vi "MicrotimeMain.vi"() -> ()   [LabVIEW 2013]
uses:
  <vilib>/vision/Pattern Matching.llb/IMAQ Curve Parameters.ctl
  <vilib>/vision/Pattern Matching.llb/IMAQ Match Range Setting.ctl
  <vilib>/vision/Image Controls.llb/IMAQ Rounding Mode.ctl
  Camera/lib/System Files/user.lib/atmcd32d.llb/Shutter_type typedef.ctl
  Camera/lib/System Files/user.lib/atmcd32d.llb/Shutter_mode typedef.ctl
  Variables/patternImg.vi
  Camera/vi/GlobalSetGetConfigureCamera.vi
  Camera/vi/ccdChipPixels.vi
  Variables/GetPicture.vi
  Variables/GlobalConAxisPI.vi
  Variables/GlobalLaserInterface.vi
  Camera/vi/StopGetPic.vi
  Camera/vi/CamDef.vi
  Camera/lib/System Files/user.lib/atmcd32d.llb/Error Code Enum typedef.ctl
panel:
  out "subarray":dbl[](array[numeric])
  in  "Settings (GeometricMatching)":T3={"Curve Parameters"={"Extraction Mode"=0, "Edge Threshold"=75, "Edge Filter Size"=1, "Min Length"=25, "Row Search Step Size"=15, "Col Search Step Size"=15, "Max Endpoint Gap"=10, "Closed"=FALSE, "Subpixel"=FALSE}, "Match Mode"={"Rotation"=TRUE, "Scale"=FALSE, "Occlusion"=TRUE, "Reserved"=FALSE, "Reserved"=FALSE, "Reserved"=FALSE}, "Range Settings"=[{"Match Constraints"=0, "Min"=0.0, "Max"=360.0}, {"Match Constraints"=2, "Min"=0.0, "Max"=25.0}], "Number of Matches"=5, "Minimum Match Score"=600.0, "SubPixel Accuracy"=FALSE, "Adv. Geometric Match Options 2"=[{"Setup Data Item"=21, "Item Value"=0.0}, {"Setup Data Item"=22, "Item Value"=1.0}]} {"Curve Parameters"."Extraction Mode" items=["Normal", "Uniform Regions"]; "Curve Parameters"."Edge Filter Size" items=["Fine", "Normal", "Contour Tracing"]; "Curve Parameters"."Max Endpoint Gap" min=0; "Curve Parameters"."Col Search Step Size" min=1 max=255 step=1; "Curve Parameters"."Row Search Step Size" min=1 max=255 step=1; "Curve Parameters"."Min Length" min=0; "Curve Parameters"."Edge Threshold" min=1 max=350 step=1; "Range Settings"."Max" format="%.2f"; "Range Settings"."Min" format="%.2f"; "Range Settings"."Match Constraints" items=["Rotation Angle (degrees)", "Scale Factor (%)", "Occlusion (%)"]; "Adv. Geometric Match Options 2"."Setup Data Item" items=["Curve Extraction Mode", "Curve Edge Threshold", "Curve Edge Filter Size", "Min Curve Length", "Curve Row Search Step Size", "Curve Col Search Step Size", "Curve Max Endpoint Gap", "Extract Closed Curves", "Enable Subpixel Curve Extraction", "Enable Correlation Score", "Enable Subpixel Accuracy", "Subpixel Iterations", "Subpixel Tolerance", "Initial Match List Length", "Enable Target Template Curve Score", "Min Match Separation Distance", "Min Match Separation Angle", "Min Match Separation Scale", "Max Match Overlap", "Enable Coarse Result", "Enable Calibration Support", "Enable Contrast Reversal", "Search Strategy", "Refinement Match Factor", "Subpixel Match Factor"]}
  in  "Tab Control":T4(tab)
  out "Histogram":i32[][](graph)
  out "Trace":i32[][](graph)=[[2, 0, 0, 1, 1, 1, 0, 0, 0, 1, 0, 1, 0, 1, 2, 2, 0, 3, 0, 2, 2, 1, 3, 1, 0, 1, 1, 1, 0, 1, 3, 1, 0, 2, 0, 1, 0, 1, 1, 0, 1, 1, 3, 1, 0, 2, 0, 1, 1, 0, 0, 2, 0, 0, 1, 1, 1, 0, 0, 1, 0, 1, 0, 0, 0, 1, 2, 1, 1, 2, 0, 2, 4, 3, 1, 1, 0, 0, 1, 1, 2, 0, 1, 1, 0, 0, 0, 1, 1, 1, 1, 3, 0, 0, 1, 0, 0, 0, 2, 1, 1, 1, 2, 1, 0, 1, 1, 0, 0, 2, 1, 1, 0, 0, 1, 1, 1, 1, 0, 2, 2, 0, 1, 2, 1, 0, 3, 0, 2, 1, 3, 0, 1, 1, 0, 0, 3, 0, 0, 0, 0, 0, 0, 0, 0, 0, 0, 0, 0, 0, 0, 0, 0, 0, 0, 0, 0, 0, 0, 0, 0, 0, 0, 0, 0, 0, 0, 0, 0, 0, 0, 0, 0, 0, 0, 0, 0, 0, 0, 0, 0, 0, 0, 0, 0, 0, 0, 0, 0, 0, 0, 0, 0, 0, 0, 0, 0, 0, 0, 0], [1, 2, 2, 0, 0, 0, 1, 2, 1, 2, 1, 1, 1, 0, 0, 0, 3, 1, 0, 1, 0, 2, 0, 2, 1, 1, 0, 0, 1, 0, 1, 2, 1, 0, 0, 0, 0, 0, 1, 0, 1, 0, 2, 0, 1, 0, 0, 0, 0, 1, 1, 3, 0, 0, 0, 2, 0, 0, 2, 0, 1, 1, 0, 0, 2, 0, 2, 1, 0, 1, 1, 0, 1, 1, 0, 0, 0, 1, 0, 0, 1, 0, 0, 0, 0, 1, 0, 1, 1, 1, 1, 0, 0, 0, 1, 1, 1, 0, 1, 0, 0, 0, 1, 1, 1, 0, 0, 1, 1, 3, 1, 0, 0, 0, 0, 0, 0, 0, 1, 2, 1, 0, 0, 0, 2, 3, 3, 2, 0, 1, 1, 1, 0, 0, 4, 0, 1, 2, 0, 0, 0, 2, 0, 0, 0, 0, 0, 0, 0, 0, 0, 0, 0, 0, 0, 0, 0, 0, 0, 0, 0, 0, 0, 0, 0, 0, 0, 0, 0, 0, 0, 0, 0, 0, 0, 0, 0, 0, 0, 0, 0, 0, 0, 0, 0, 0, 0, 0, 0, 0, 0, 0, 0, 0, 0, 0, 0, 0, 0, 0], [2, 2, 0, 1, 2, 0, 1, 0, 2, 3, 1, 0, 1, 0, 1, 0, 0, 0, 0, 2, 1, 0, 0, 2, 2, 0, 0, 0, 3, 0, 0, 2, 2, 2, 0, 3, 0, 3, 1, 3, 1, 3, 1, 0, 3, 1, 3, 3, 1, 1, 1, 1, 2, 0, 1, 0, 1, 1, 1, 3, 0, 2, 3, 1, 1, 1, 0, 1, 0, 1, 2, 3, 1, 2, 1, 3, 0, 2, 0, 2, 0, 1, 0, 2, 2, 1, 1, 3, 1, 2, 1, 1, 1, 3, 0, 0, 0, 0, 1, 1, 1, 0, 1, 0, 2, 1, 1, 0, 1, 0, 1, 2, 2, 2, 2, 0, 1, 0, 0, 0, 1, 1, 2, 0, 0, 1, 5, 2, 2, 0, 2, 0, 2, 2, 2, 0, 1, 0, 6, 0, 0, 0, 0, 0, 0, 0, 0, 0, 0, 0, 0, 0, 0, 0, 0, 0, 0, 0, 0, 0, 0, 0, 0, 0, 0, 0, 0, 0, 0, 0, 0, 0, 0, 0, 0, 0, 0, 0, 0, 0, 0, 0, 0, 0, 0, 0, 0, 0, 0, 0, 0, 0, 0, 0, 0, 0, 0, 0, 0, 0], [0, 0, 1, 0, 1, 1, 0, 0, 0, 1, 1, 0, 1, 0, 0, 0, 0, 0, 2, 0, 0, 0, 0, 2, 0, 0, 0, 1, 1, 2, 1, 1, 1, 2, 1, 0, 0, 3, 0, 1, 1, 0, 0, 0, 0, 1, 0, 0, 2, 1, 0, 0, 1, 1, 1, 2, 2, 0, 1, 0, 0, 1, 0, 1, 1, 0, 0, 2, 1, 1, 2, 1, 1, 0, 0, 0, 0, 2, 1, 0, 0, 0, 0, 1, 0, 1, 0, 0, 0, 0, 1, 0, 0, 0, 0, 1, 0, 1, 1, 1, 0, 2, 3, 1, 1, 0, 1, 1, 1, 0, 1, 0, 0, 1, 1, 0, 2, 0, 0, 0, 0, 3, 0, 0, 0, 0, 0, 0, 0, 0, 1, 0, 2, 0, 0, 0, 1, 2, 2, 0, 1, 0, 0, 0, 0, 0, 0, 0, 0, 0, 0, 0, 0, 0, 0, 0, 0, 0, 0, 0, 0, 0, 0, 0, 0, 0, 0, 0, 0, 0, 0, 0, 0, 0, 0, 0, 0, 0, 0, 0, 0, 0, 0, 0, 0, 0, 0, 0, 0, 0, 0, 0, 0, 0, 0, 0, 0, 0, 0, 0]]
  out "CCD":i32[][](graph)
  out "Image Out":T5(plugin-control)
  out "Image Number":u32
  out "acquired FPS":dbl
  out "Image":i32[][](graph)
  out "AM image":T5(plugin-control)
  out "Number of Particles":i32
  out "Auto Measure Points":i32
  out "NxtAutMesPoint":i32
  out "Pattern":dbl[][](array[numeric])
  out "X Steps":dbl
  out "3dAbelFcs":bool=TRUE
  out "Y Steps":dbl
  out "Z Steps":dbl
  out "concatenated string":string
  out "Global Stop":bool=TRUE
  out "Stop Measurement":bool
  in  "DeviceTabs":T6(tab)
  in  "WS File Tree":string(tree)
  out "Workspace":path=path "X:/MTusers/Christoph/2011-02-01 Andi/2011-02-01.msw"
  in  "New MSW":bool
  in  "Open MSW":bool
  in  "Sample description":string
  in  "Save Files":bool=TRUE
  out "Last Image File No":i32=-1
  in  "Get Position":bool
  in  "Move Stage":bool
  in  "X-Position":dbl=48.0021 caption="X" min=0.0 max=200.0 step=0.1 format="%1.3f um"
  in  "Y-Position":dbl=19.9997 caption="Y" min=0.0 max=200.0 step=0.1 format="%1.3f um"
  in  "Z-Position":dbl=69.999 caption="Z" min=0.0 max=200.0 step=0.1 format="%1.3f um"
  out "x-position":dbl format="%.3f"
  out "y-position":dbl format="%.3f"
  out "z-position":dbl format="%.3f"
  in  "CFD Settings":T7={"Sync Level"=15, "Sync ZeroX"=0, "Sync Offset"=0, "Chan Settings"=[{"CHx Level"=50, "CHx ZeroX"=10, "CHx Offset"=-22150}, {"CHx Level"=50, "CHx ZeroX"=10, "CHx Offset"=-21850}, {"CHx Level"=75, "CHx ZeroX"=10, "CHx Offset"=-6000}, {"CHx Level"=75, "CHx ZeroX"=10, "CHx Offset"=-5700}]}
  in  "Laser  Profile":string="1"
  in  "Auto Exposure::Mode":u32(ring) items=["Relative"=0, "Ignored"=5]
  in  "Brightness::Mode":u32(ring) items=["Relative"=0, "Ignored"=5]
  in  "Gain::Mode":u32(ring) items=["Absolute"=1, "Auto"=3, "Relative"=0, "Ignored"=5]
  in  "Gamma::Mode":u32(ring)=2 items=["Relative"=0, "Off"=2, "Ignored"=5]
  in  "Shutter::Mode":u32(ring) items=["Auto"=3, "Relative"=0, "Ignored"=5]
  in  "Trigger::Trigger Activation":u32(ring) items=["Level Low", "Level High"]
  in  "Trigger::Trigger Mode":u32(ring)=16 items=["Mode 0"=0, "Mode 1"=1, "Mode 15"=15, "Off"=16]
  in  "Trigger Delay::Mode":u32(ring)=2 items=["Absolute"=1, "Relative"=0, "Off"=2, "Ignored"=5]
  in  "Brightness::Value":dbl=16.0 min=0.0 max=1023.0 step=1.0
  in  "Shutter::Value":dbl=436.0 min=1.0 max=4095.0 step=1.0
  in  "Auto Exposure::Value":dbl=125.0 min=50.0 max=205.0 step=1.0
  in  "Gain::Value":dbl min=0.0 max=680.0 step=1.0
  in  "Trigger::Trigger Parameter":u32 max=0
  in  "Get Temperature":bool
  in  "SET CCD":bool
  in  "OPEN SHUTER":bool
  in  "Close":bool
  in  "Gain":bool
  in  "Start":bool
  in  "Stop":bool
  in  "Exposure":bool
  in  "Set Temperature":bool
  in  "PI SystemNumber":i32=1
  in  "Image Measurent Parameters":T8
  in  "Measurement Tab Control":T9(tab)
  in  "SCANNER EMERGENCY":bool
  in  "Stop Program":bool
  out "Task":T10(ring)
  in  "Point Defocussed Cam":bool
  in  "Adjustment":bool
  in  "Laser pulse duration":i32[](array[numeric]) min=2 max=100000 step=1 format="%d µs"
  in  "Measurement Time":i32=60 min=10 format="%.0d s"
  in  "Point Measurement":bool
  out "Counts":u32[](array[numeric])
  in  "Axis":enum32{"x-y", "x-z", "y-x", "y-z", "z-x", "z-y"}(ring)
  in  "Picture size 2":dbl=50.0 min=0.1 max=200.0 format="%1.1f um"
  in  "Picture size":dbl=50.0 min=0.1 max=200.0 format="%1.1f um"
  in  "Pixel time":dbl=1.0 min=0.1 max=10.0 step=0.1 format="%.1f ms"
  in  "Resolution":dbl=1.0 min=0.05 max=10.0 step=0.05 format="%.2f µm"
  out "Measure. time":dbl format="%7.1f s"
  in  "Aquire Image":bool
  out "y":i16=500
  out "x":i16=500
  in  "Save Color Image":bool
  in  "Cam (Defocused)":bool
  in  "How long?":bool
  out "Estimated Time (h)":dbl
  in  "Mesaurement Time (Sec) / Step":dbl
  in  "Start 3D FCS Abel Scan":bool
  in  "FCS Point Measurement":bool
  in  "Z Stepsize":dbl
  in  "Y Stepsize":dbl
  in  "X Stepsize":dbl
  in  "Z End":dbl
  in  "Y End":dbl
  in  "X End":dbl
  in  "Z Start":dbl
  in  "Y Start":dbl
  in  "X Start":dbl
  in  "Manual":bool
  in  "Find Mols":bool
  in  "Filter":bool=TRUE
  in  "Remove Outliers":i32=10
  in  "Exclude / Include X":bool
  in  "X Start 2":dbl
  in  "X End 2":dbl
  in  "Exclude / Include Y":bool
  in  "Y Start 2":dbl
  in  "Y End 2":dbl
  in  "Measurement Parameter 1":T11 items=["Center of Mass X", "Center of Mass Y", "First Pixel X", "First Pixel Y", "Bounding Rect Left", "Bounding Rect Top", "Bounding Rect Right", "Bounding Rect Bottom", "Max Feret Diameter Start X", "Max Feret Diameter Start Y", "Max Feret Diameter End X", "Max Feret Diameter End Y", "Max Horiz. Segment Length Left", "Max Horiz. Segment Length Right", "Max Horiz. Segment Length Row", "-", "Bounding Rect Width", "Bounding Rect Height", "Bounding Rect Diagonal", "Perimeter", "Convex Hull Perimeter", "Holes' Perimeter", "Max Feret Diameter", "Equivalent Ellipse Major Axis", "Equivalent Ellipse Minor Axis", "Equivalent Ellipse Minor Axis (Feret)", "Equivalent Rect Long Side", "Equivalent Rect Short Side", "Equivalent Rect Diagonal", "Equivalent Rect Short Side (Feret)", "Average Horiz. Segment Length", "Average Vert. Segment Length", "Hydraulic Radius", "Waddel Disk Diameter", "-", "Area", "Holes' Area", "Particle & Holes' Area", "Convex Hull Area", "Image Area", "-", "Number of Holes", "Number of Horiz. Segments", "Number of Vert. Segments", "-", "Orientation", "Max Feret Diameter Orientation", "-", "% Area/Image Area", "% Area/(Particle & Holes' Area)", "Ratio of Equivalent Ellipse Axes", "Ratio of Equivalent Rect Sides", "-", "Elongation Factor", "Compactness Factor", "Heywood Circularity Factor", "Type Factor", "-", "Sum X", "Sum Y", "Sum XX", "Sum XY", "Sum YY", "Sum XXX", "Sum XXY", "Sum XYY", "Sum YYY", "-", "Moment of Inertia XX", "Moment of Inertia XY", "Moment of Inertia YY", "Moment of Inertia XXX", "Moment of Inertia XXY", "Moment of Inertia XYY", "Moment of Inertia YYY", "Norm. Moment of Inertia XX", "Norm. Moment of Inertia XY", "Norm. Moment of Inertia YY", "Norm. Moment of Inertia XXX", "Norm. Moment of Inertia XXY", "Norm. Moment of Inertia XYY", "Norm. Moment of Inertia YYY", "Hu Moment 1", "Hu Moment 2", "Hu Moment 3", "Hu Moment 4", "Hu Moment 5", "Hu Moment 6", "Hu Moment 7"]
  in  "Range Lower Value Par 1":dbl
  in  "Range Upper Value  Par 1":dbl
  in  "Ex/In Par 1":bool
  in  "Measurement Parameter 2":T11 items=["Center of Mass X", "Center of Mass Y", "First Pixel X", "First Pixel Y", "Bounding Rect Left", "Bounding Rect Top", "Bounding Rect Right", "Bounding Rect Bottom", "Max Feret Diameter Start X", "Max Feret Diameter Start Y", "Max Feret Diameter End X", "Max Feret Diameter End Y", "Max Horiz. Segment Length Left", "Max Horiz. Segment Length Right", "Max Horiz. Segment Length Row", "-", "Bounding Rect Width", "Bounding Rect Height", "Bounding Rect Diagonal", "Perimeter", "Convex Hull Perimeter", "Holes' Perimeter", "Max Feret Diameter", "Equivalent Ellipse Major Axis", "Equivalent Ellipse Minor Axis", "Equivalent Ellipse Minor Axis (Feret)", "Equivalent Rect Long Side", "Equivalent Rect Short Side", "Equivalent Rect Diagonal", "Equivalent Rect Short Side (Feret)", "Average Horiz. Segment Length", "Average Vert. Segment Length", "Hydraulic Radius", "Waddel Disk Diameter", "-", "Area", "Holes' Area", "Particle & Holes' Area", "Convex Hull Area", "Image Area", "-", "Number of Holes", "Number of Horiz. Segments", "Number of Vert. Segments", "-", "Orientation", "Max Feret Diameter Orientation", "-", "% Area/Image Area", "% Area/(Particle & Holes' Area)", "Ratio of Equivalent Ellipse Axes", "Ratio of Equivalent Rect Sides", "-", "Elongation Factor", "Compactness Factor", "Heywood Circularity Factor", "Type Factor", "-", "Sum X", "Sum Y", "Sum XX", "Sum XY", "Sum YY", "Sum XXX", "Sum XXY", "Sum XYY", "Sum YYY", "-", "Moment of Inertia XX", "Moment of Inertia XY", "Moment of Inertia YY", "Moment of Inertia XXX", "Moment of Inertia XXY", "Moment of Inertia XYY", "Moment of Inertia YYY", "Norm. Moment of Inertia XX", "Norm. Moment of Inertia XY", "Norm. Moment of Inertia YY", "Norm. Moment of Inertia XXX", "Norm. Moment of Inertia XXY", "Norm. Moment of Inertia XYY", "Norm. Moment of Inertia YYY", "Hu Moment 1", "Hu Moment 2", "Hu Moment 3", "Hu Moment 4", "Hu Moment 5", "Hu Moment 6", "Hu Moment 7"]
  in  "Range Lower Value Par 2":dbl
  in  "Range Upper Value Par 2":dbl
  in  "Ex/In Par 2":bool
  in  "Square/Hexa":bool=TRUE
  in  "Connectivity 4/8":bool
  in  "Auto Defocussed Cam":bool
  in  "Autopoint-Autofocus Z":bool=TRUE
  in  "Auto Measurement Time (ms)":i32=60 caption="Measurement Time (s)" min=10
  out "Auto Meas Progress":i32(slide) caption="Point 2 / 2" scale=0.0..2.0
  in  "Auto Meas":bool
  out "Active pt3":path
  out "Buffer Overrun":bool
  out "Running":bool
  # "Range"
  # "Scanner Position"
  # "Point Measurement Settings"
  # "Start Experiment"
  # "Estimated Mesaurement Time"
  # "Image Scan Settings"
  # "Save as png"
  # "Pixel"
  # "Define the 3D Space and Stepwith of your Experiment"
  # "Time of the Experiment"
  # "Check What to Mesaure"
  # "Start Your Experiment here"
  # "Lifetime Mesaurement Time on each Position"
  # "Define Search Area"
  # "Define Detection Parameters"
  # "Exact Matching"
  # "Show Progress"
  # "Automated Mesaurement on Single Molecule Coordinates on the  2D Frame"
  # "Start Your Experiment here"
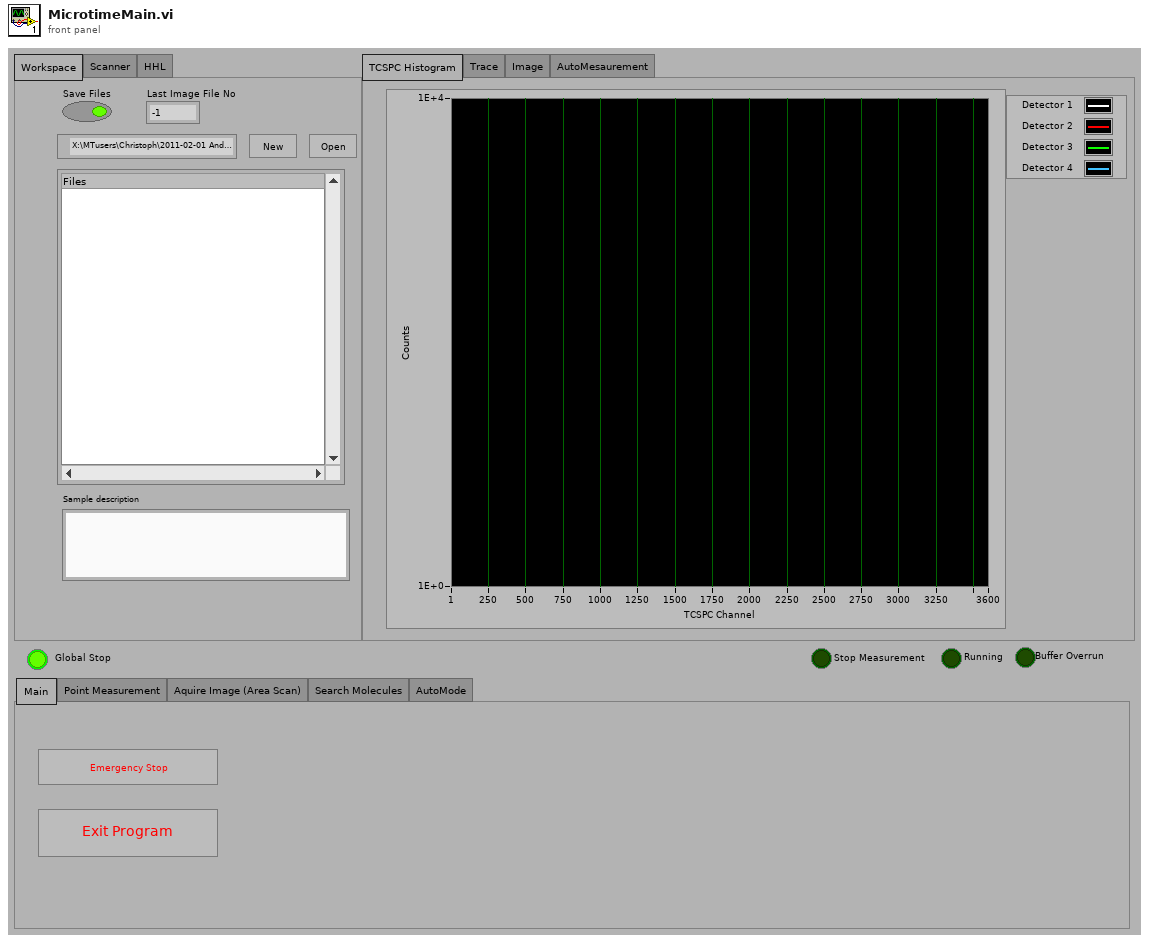
[diagram p1: front panel]
types:
  T1 = typedef "IMAQ Curve Parameters.ctl" = cluster{"Extraction Mode":u32, "Edge Threshold":i32, "Edge Filter Size":u32, "Min Length":i32, "Row Search Step Size":i32, "Col Search Step Size":i32, "Max Endpoint Gap":i32, "Closed":bool, "Subpixel":bool}
  T2 = typedef "IMAQ Match Range Setting.ctl" = cluster{"Match Constraints":u32, "Min":dbl, "Max":dbl}
  T3 = cluster{"Curve Parameters":T1, "Match Mode":cluster{"Rotation":bool, "Scale":bool, "Occlusion":bool, "Reserved":bool, "Reserved":bool, "Reserved":bool}, "Range Settings":T2[], "Number of Matches":i32, "Minimum Match Score":sgl, "SubPixel Accuracy":bool, "Adv. Geometric Match Options 2":cluster{"Setup Data Item":u16, "Item Value":dbl}[]}
  T4 = enum32{"TCSPC Histogram", "Trace", "CCD", "Backreflection", "Image", "AutoMesaurement"}
  T5 = typedef "IMAQ Image.ctl" = refnum<image>
  T6 = enum32{"Workspace", "Scanner", "HHL", "Video", "CCD"}
  T7 = cluster{"Sync Level":i32, "Sync ZeroX":i32, "Sync Offset":i32, "Chan Settings":cluster{"CHx Level":i32, "CHx ZeroX":i32, "CHx Offset":i32}[]}
  T8 = cluster{"Position":cluster{"X-Position":dbl, "Y-Position":dbl, "Z-Position":dbl}, "Axis 1 Pixels":dbl, "Axis 2 Pixels":dbl, "Axis":i32, "Resolution":dbl, "PixelTime":dbl, "Laser pulses":i32}
  T9 = enum32{"Main ", "Point Measurement", "Aquire Image (Area Scan)", "3D Grid FCS CCD", "Search Molecules", "AutoMode"}
  T10 = enum16{"No Measurement", "Aquire Image", "Point Measurement", "Multi Measurement", "Save Color Image", "Find Single Mol.", "Auto Measurement Control", "Auto Point", "Aquire Line Scan", "Grid Measurement", "Trapping", "Move Scanner"}
  T11 = typedef "Particle Parameters" = i32
  T12 = cluster{"Dev":i32, "SerNo":string, "HW_Model":string, "HW_Partno":string}[]
  T13 = typedef "Shutter_type typedef.ctl" = enum16{"TTL Low", "TTL High"}
  T14 = typedef "Shutter_mode typedef.ctl" = enum16{"Auto", "Open", "Close"}
  T15 = typedef "Error Code Enum typedef.ctl" = enum32{"N/A (0)", "DRV_ERROR_CODES", "DRV_SUCCESS", "DRV_VXDNOTINSTALLED", "DRV_ERROR_SCAN", "DRV_ERROR_CHECK_SUM", "DRV_ERROR_FILELOAD", "DRV_UNKNOWN_FUNC", "DRV_ERROR_VXD_INIT", "DRV_ERROR_ADDRESS", "DRV_ERROR_PAGELOCK", "DRV_ERROR_PAGEUNLOCK", "DRV_ERROR_BOARDTEST", "DRV_ERROR_ACK", "DRV_ERROR_UP_FIFO", "DRV_ERROR_PATTERN", "N/A (16)", "DRV_ACQUISITION_ERRORS", "DRV_ACQ_BUFFER", "DRV_ACQ_DOWNFIFO_FULL", "DRV_PROC_UNKONWN_INSTRUCTION", "DRV_ILLEGAL_OP_CODE", "DRV_KINETIC_TIME_NOT_MET", "DRV_ACCUM_TIME_NOT_MET", "DRV_NO_NEW_DATA", "N/A (25)", "DRV_SPOOLERROR", "N/A (27)", "N/A (28)", "N/A (29)", "N/A (30)", "N/A (31)", "N/A (32)", "DRV_TEMPERATURE_CODES", "DRV_TEMPERATURE_OFF", "DRV_TEMPERATURE_NOT_STABILIZED", "DRV_TEMPERATURE_STABILIZED", "DRV_TEMPERATURE_NOT_REACHED", "DRV_TEMPERATURE_OUT_RANGE", "DRV_TEMPERATURE_NOT_SUPPORTED", "DRV_TEMPERATURE_DRIFT", "N/A (41)", "N/A (42)", "N/A (43)", "N/A (44)", "N/A (45)", "N/A (46)", "N/A (47)", "N/A (48)", "DRV_GENERAL_ERRORS", "DRV_INVALID_AUX", "DRV_COF_NOTLOADED", "DRV_FPGAPROG", "DRV_FLEXERROR", "DRV_GPIBERROR", "N/A (55)", "N/A (56)", "N/A (57)", "N/A (58)", "N/A (59)", "N/A (60)", "N/A (61)", "N/A (62)", "N/A (63)", "DRV_DATATYPE", "DRV_DRIVER_ERRORS", "DRV_P1INVALID", "DRV_P2INVALID", "DRV_P3INVALID", "DRV_P4INVALID", "DRV_INIERROR", "DRV_COFERROR", "DRV_ACQUIRING", "DRV_IDLE", "DRV_TEMPCYCLE", "DRV_NOT_INITIALIZED", "DRV_P5INVALID", "DRV_P6INVALID", "DRV_INVALID_MODE", "DRV_INVALID_FILTER", "DRV_I2CERRORS", "DRV_I2CDEVNOTFOUND", "DRV_I2CTIMEOUT", "DRV_P7INVALID", "N/A (84)", "N/A (85)", "N/A (86)", "N/A (87)", "N/A (88)", "N/A (89)", "DRV_IOCERROR", "DRV_VRMVERSIONERROR"}
  T16 = cluster{"X-Position":dbl, "Y-Position":dbl, "Z-Position":dbl}
  T17 = enum16{"No Measurement", "Aquire Image", "Point Measurement", "Multi Measurement", "Save Color Image"}
  T18 = enum16{"No Measurement", "Aquire Image", "Point Measurement", "Multi Measurement", "Save Color Image", "Find Single Mol.", "Auto Measurement Control", "Auto Point"}
  T19 = enum16{"No Measurement", "Aquire Image", "Point Measurement", "Multi Measurement", "Save Color Image", "Find Single Mol."}
  T20 = enum16{"Get (Default)", "Set Workspace", "Append File", "Change Comment"}
  T21 = cluster{"File No":i32, "File Path":path, "Parent File":i32, "File Type":enum16{"unknown", "pt3 File", "png Image", "bmp Image"}, "Measurement Type":enum16{"not a pt3 File", "Image File", "Point Measurement", "Auto Point", "Line Scan", "Grid Scan"}, "Upper Left":cluster{"x-Position":dbl, "y-Position":dbl, "z-Position":dbl}, "Pixels":dbl[], "Resolution":dbl, "Scan Axis":enum32{"x-y", "x-z", "y-x", "y-z", "z-x", "z-y"}, "PixelTime":dbl}[]
  T22 = cluster{"File No":i32, "File Path":path, "Parent File":i32, "File Type":enum16{"unknown", "pt3 File", "png Image", "bmp Image"}, "Measurement Type":enum16{"not a pt3 File", "Image File", "Point Measurement", "Auto Point", "Line Scan", "Grid Scan"}, "Upper Left":cluster{"x-Position":dbl, "y-Position":dbl, "z-Position":dbl}, "Pixels":i32[], "Scan Axis":enum32{"x-y", "x-z", "y-x", "y-z", "z-x", "z-y"}, "Resolution":dbl, "PixelTime":dbl}[]
  T23 = cluster{"File No":i32, "File Path":path, "Parent File":i32, "File Type":enum16{"unknown", "pt3 File", "png Image", "bmp Image"}, "Measurement Type":enum16{"not a pt3 File", "Image File", "Point Measurement", "Auto Point", "Line Scan", "Grid Scan"}, "Upper Left":cluster{"x-Position":dbl, "y-Position":dbl, "z-Position":dbl}, "Pixels":i32[], "Resolution":dbl, "Scan Axis":enum32{"x-y", "x-z", "y-z"}, "PixelTime":dbl}[]
  T24 = cluster{"Files in Workspace[0]":cluster{"File No":i32, "File Path":path, "Parent File":i32, "File Type":enum16{"unknown", "pt3 File", "png Image", "bmp Image"}, "Measurement Type":enum16{"not a pt3 File", "Image File", "Point Measurement", "Auto Point", "Line Scan", "Grid Scan"}, "Upper Left":cluster{"x-Position":dbl, "y-Position":dbl, "z-Position":dbl}, "Pixels":i32[], "Scan Axis":enum32{"x-y", "x-z", "y-x", "y-z", "z-x", "z-y"}, "Resolution":dbl, "PixelTime":dbl}, "Files in Workspace[1]":cluster{"File No":i32, "File Path":path, "Parent File":i32, "File Type":enum16{"unknown", "pt3 File", "png Image", "bmp Image"}, "Measurement Type":enum16{"not a pt3 File", "Image File", "Point Measurement", "Auto Point", "Line Scan", "Grid Scan"}, "Upper Left":cluster{"x-Position":dbl, "y-Position":dbl, "z-Position":dbl}, "Pixels":i32[], "Scan Axis":enum32{"x-y", "x-z", "y-x", "y-z", "z-x", "z-y"}, "Resolution":dbl, "PixelTime":dbl}, "Files in Workspace[2]":cluster{"File No":i32, "File Path":path, "Parent File":i32, "File Type":enum16{"unknown", "pt3 File", "png Image", "bmp Image"}, "Measurement Type":enum16{"not a pt3 File", "Image File", "Point Measurement", "Auto Point", "Line Scan", "Grid Scan"}, "Upper Left":cluster{"x-Position":dbl, "y-Position":dbl, "z-Position":dbl}, "Pixels":i32[], "Scan Axis":enum32{"x-y", "x-z", "y-x", "y-z", "z-x", "z-y"}, "Resolution":dbl, "PixelTime":dbl}, "Files in Workspace[3]":cluster{"File No":i32, "File Path":path, "Parent File":i32, "File Type":enum16{"unknown", "pt3 File", "png Image", "bmp Image"}, "Measurement Type":enum16{"not a pt3 File", "Image File", "Point Measurement", "Auto Point", "Line Scan", "Grid Scan"}, "Upper Left":cluster{"x-Position":dbl, "y-Position":dbl, "z-Position":dbl}, "Pixels":i32[], "Scan Axis":enum32{"x-y", "x-z", "y-x", "y-z", "z-x", "z-y"}, "Resolution":dbl, "PixelTime":dbl}, "Files in Workspace[4]":cluster{"File No":i32, "File Path":path, "Parent File":i32, "File Type":enum16{"unknown", "pt3 File", "png Image", "bmp Image"}, "Measurement Type":enum16{"not a pt3 File", "Image File", "Point Measurement", "Auto Point", "Line Scan", "Grid Scan"}, "Upper Left":cluster{"x-Position":dbl, "y-Position":dbl, "z-Position":dbl}, "Pixels":i32[], "Scan Axis":enum32{"x-y", "x-z", "y-x", "y-z", "z-x", "z-y"}, "Resolution":dbl, "PixelTime":dbl}, "Files in Workspace[5]":cluster{"File No":i32, "File Path":path, "Parent File":i32, "File Type":enum16{"unknown", "pt3 File", "png Image", "bmp Image"}, "Measurement Type":enum16{"not a pt3 File", "Image File", "Point Measurement", "Auto Point", "Line Scan", "Grid Scan"}, "Upper Left":cluster{"x-Position":dbl, "y-Position":dbl, "z-Position":dbl}, "Pixels":i32[], "Scan Axis":enum32{"x-y", "x-z", "y-x", "y-z", "z-x", "z-y"}, "Resolution":dbl, "PixelTime":dbl}, "Files in Workspace[6]":cluster{"File No":i32, "File Path":path, "Parent File":i32, "File Type":enum16{"unknown", "pt3 File", "png Image", "bmp Image"}, "Measurement Type":enum16{"not a pt3 File", "Image File", "Point Measurement", "Auto Point", "Line Scan", "Grid Scan"}, "Upper Left":cluster{"x-Position":dbl, "y-Position":dbl, "z-Position":dbl}, "Pixels":i32[], "Scan Axis":enum32{"x-y", "x-z", "y-x", "y-z", "z-x", "z-y"}, "Resolution":dbl, "PixelTime":dbl}, "Files in Workspace[7]":cluster{"File No":i32, "File Path":path, "Parent File":i32, "File Type":enum16{"unknown", "pt3 File", "png Image", "bmp Image"}, "Measurement Type":enum16{"not a pt3 File", "Image File", "Point Measurement", "Auto Point", "Line Scan", "Grid Scan"}, "Upper Left":cluster{"x-Position":dbl, "y-Position":dbl, "z-Position":dbl}, "Pixels":i32[], "Scan Axis":enum32{"x-y", "x-z", "y-x", "y-z", "z-x", "z-y"}, "Resolution":dbl, "PixelTime":dbl}, "Files in Workspace[8]":cluster{"File No":i32, "File Path":path, "Parent File":i32, "File Type":enum16{"unknown", "pt3 File", "png Image", "bmp Image"}, "Measurement Type":enum16{"not a pt3 File", "Image File", "Point Measurement", "Auto Point", "Line Scan", "Grid Scan"}, "Upper Left":cluster{"x-Position":dbl, "y-Position":dbl, "z-Position":dbl}, "Pixels":i32[], "Scan Axis":enum32{"x-y", "x-z", "y-x", "y-z", "z-x", "z-y"}, "Resolution":dbl, "PixelTime":dbl}}
  T25 = typedef "LVPoint32TypeDef.ctl" = cluster{"Horizontal":i32, "Vertical":i32}
  T26 = cluster{"Shift":bool, "Ctrl":bool, "Alt":bool, "Cmd":bool, "Opt":bool}
  T27 = enum16{"No Measurement", "Aquire Image", "Point Measurement", "Multi Measurement", "Save Color Image", "Find Single Mol.", "Auto Measurement Control", "Auto Point", "Aquire Line Scan", "Grid Measurement"}
  T28 = enum16{"none", "fast axis", "slow axis", "both axis", ""}
  T29 = enum16{"none", "fast axis", "slow axis", "both", ""}
  T30 = enum16{"target position", "relative position", "actual position", "position error"}
  T31 = enum16{"not a pt3 File", "Image File", "Point Measurement", "Auto Point"}
  T32 = enum16{"unknown", "pt3 File", "png Image", "bmp Image"}
  T33 = typedef "IMAQ Rounding Mode.ctl" = enum16{"Optimize", "Truncate"}
  T34 = cluster{"Measurement Parameter":T11, "Range Lower Value":dbl, "Range Upper Value":dbl, "Range":bool, "Measurement Type":bool}[]
  T35 = enum16{"not a pt3 File", "Image File", "Point Measurement", "Auto Point", "Line Scan"}
  T36 = cluster{"Dev":i32, "SerNo":string, "HW_Model":string, "HW_Partno":string}
  T37 = cluster{"Comment":string, "Binning":i32, "Offset":i32, "AcquisitionTime (ms)":i32, "HardwareSerial":i32, "SyncDivider":i32, "Resolution (ps)":dbl, "CFD Settings":cluster{"Sync Level":i32, "Sync ZeroX":i32, "Sync Offset":i32, "Chan Settings":cluster{"CHx Level":i32, "CHx ZeroX":i32, "CHx Offset":i32}[]}, "ModuleInfo":cluster{"modelcode":i32, "versioncode":i32}[], "BaseResolution (ps)":dbl, "RefClockSource":i32, "ChanInfo":cluster{"CHx Level":i32, "CHx ZeroX":i32, "CHx Offset":i32, "CHx modidx":i32}[], "SyncRate":i32, "InputsEnabled":i64}
  T38 = cluster{"Dimensions":i32, "Time Per Pixel [ms]":dbl, "Acceleration":i32, "Pattern":i32, "X0":sgl, "Y0":sgl, "Z0":dbl, "PixX":i32, "PixY":i32, "PixResol":sgl, "TStartTo":sgl, "TStoptTo":sgl, "TStartFro":sgl, "TStopFro":sgl}
  T39 = cluster{"InpRateFilePos":i64, "StopAfterFilePos":i64}
  T40 = cluster{"File No":i32, "File Path":path, "Parent File":i32, "File Type":enum16{"unknown", "pt3 File", "png Image", "bmp Image"}, "Measurement Type":enum16{"not a pt3 File", "Image File", "Point Measurement", "Auto Point", "Line Scan", "Grid Scan"}, "Upper Left":cluster{"x-Position":dbl, "y-Position":dbl, "z-Position":dbl}, "Pixels":i32[], "Scan Axis":enum32{"x-y", "x-z", "y-z"}, "Resolution":dbl, "PixelTime":dbl}
  T41 = enum16{"not a pt3 File", "Image File", "Point Measurement", "Auto Point", "Line Scan", "Grid Scan"}
  T42 = cluster{"Ident":string, "Format Version":string, "Creator Name":string, "Creator Version":string, "File Time":string, "Comment":string, "Laser":i32, "Binning":i32, "Offset":i32, "AcquisitionTime (ms)":i32, "HardwareSerial":i32, "SyncDivider":i32, "Resolution (ps)":dbl, "Rates":dbl[], "SyncRate":dbl, "CFD Settings":cluster{"Sync Level":i32, "Sync ZeroX":i32, "Sync Offset":i32, "Chan Settings":cluster{"CHx Level":i32, "CHx ZeroX":i32, "CHx Offset":i32}[]}}
  T43 = cluster{"x-Position":dbl, "y-Position":dbl, "z-Position":dbl}
  T44 = typedef "Image Type" = u32
  T45 = cluster{"MesaurementSelection[0]":cluster{"Measurement Parameter":T11, "Range Lower Value":dbl, "Range Upper Value":dbl, "Range":bool, "Measurement Type":bool}, "MesaurementSelection[1]":cluster{"Measurement Parameter":T11, "Range Lower Value":dbl, "Range Upper Value":dbl, "Range":bool, "Measurement Type":bool}, "MesaurementSelection[2]":cluster{"Measurement Parameter":T11, "Range Lower Value":dbl, "Range Upper Value":dbl, "Range":bool, "Measurement Type":bool}, "MesaurementSelection[3]":cluster{"Measurement Parameter":T11, "Range Lower Value":dbl, "Range Upper Value":dbl, "Range":bool, "Measurement Type":bool}, "MesaurementSelection[4]":cluster{"Measurement Parameter":T11, "Range Lower Value":dbl, "Range Upper Value":dbl, "Range":bool, "Measurement Type":bool}, "MesaurementSelection[5]":cluster{"Measurement Parameter":T11, "Range Lower Value":dbl, "Range Upper Value":dbl, "Range":bool, "Measurement Type":bool}, "MesaurementSelection[6]":cluster{"Measurement Parameter":T11, "Range Lower Value":dbl, "Range Upper Value":dbl, "Range":bool, "Measurement Type":bool}, "MesaurementSelection[7]":cluster{"Measurement Parameter":T11, "Range Lower Value":dbl, "Range Upper Value":dbl, "Range":bool, "Measurement Type":bool}, "MesaurementSelection[8]":cluster{"Measurement Parameter":T11, "Range Lower Value":dbl, "Range Upper Value":dbl, "Range":bool, "Measurement Type":bool}}
  T46 = cluster{"Measurement Parameter":T11, "Range Lower Value":dbl, "Range Upper Value":dbl, "Range":bool, "Measurement Type":bool}
  T47 = typedef "IMAQ GM Match Report.ctl" = cluster{"Position":cluster{"x":sgl, "y":sgl}, "Angle":sgl, "Scale":sgl, "Score":sgl, "Bounding Box":cluster{"x":sgl, "y":sgl}[], "Contrast Reversed":bool, "Occlusion %":sgl, "Template Target Curve Score":sgl, "Target Template Curve Score":sgl, "Correlation Score":sgl}
  T48 = typedef "IMAQ Point" = cluster{"X":sgl, "Y":sgl}
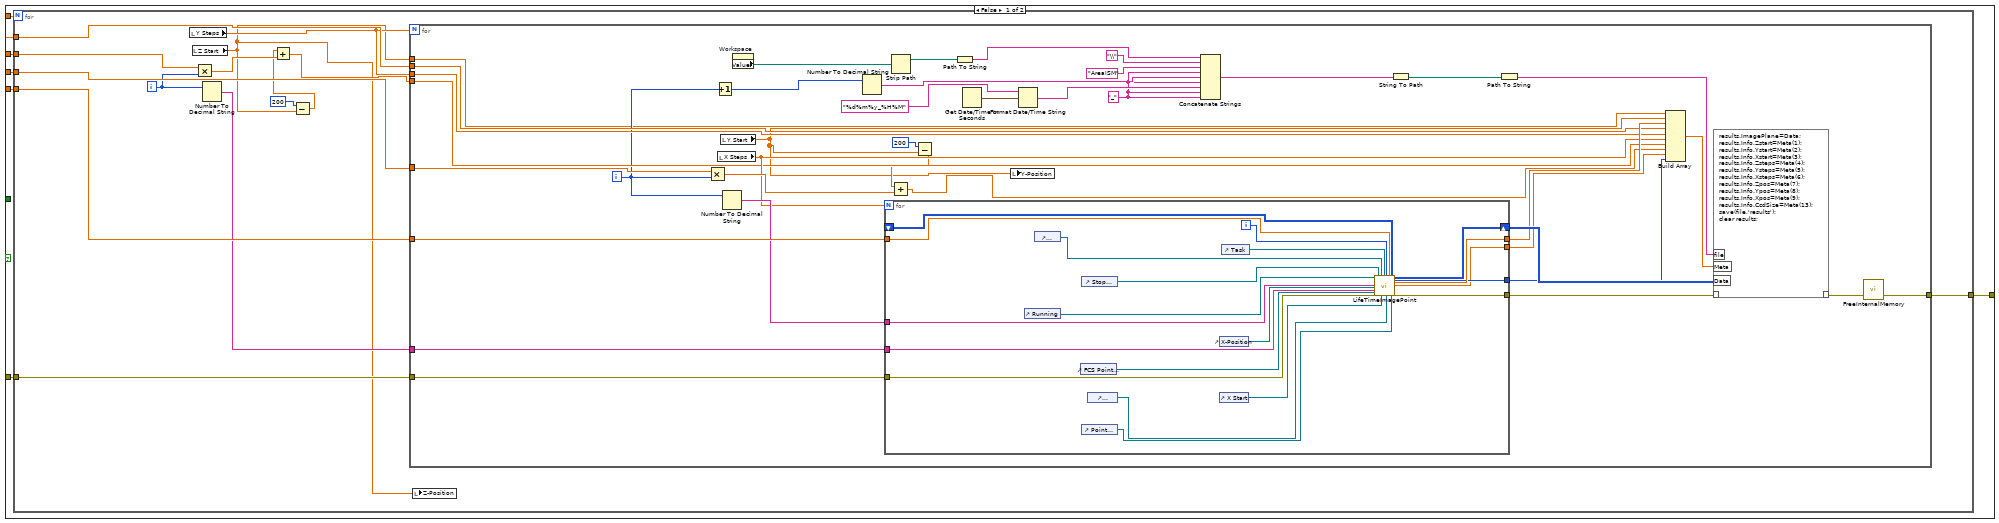
[diagram p5: hidden frame]
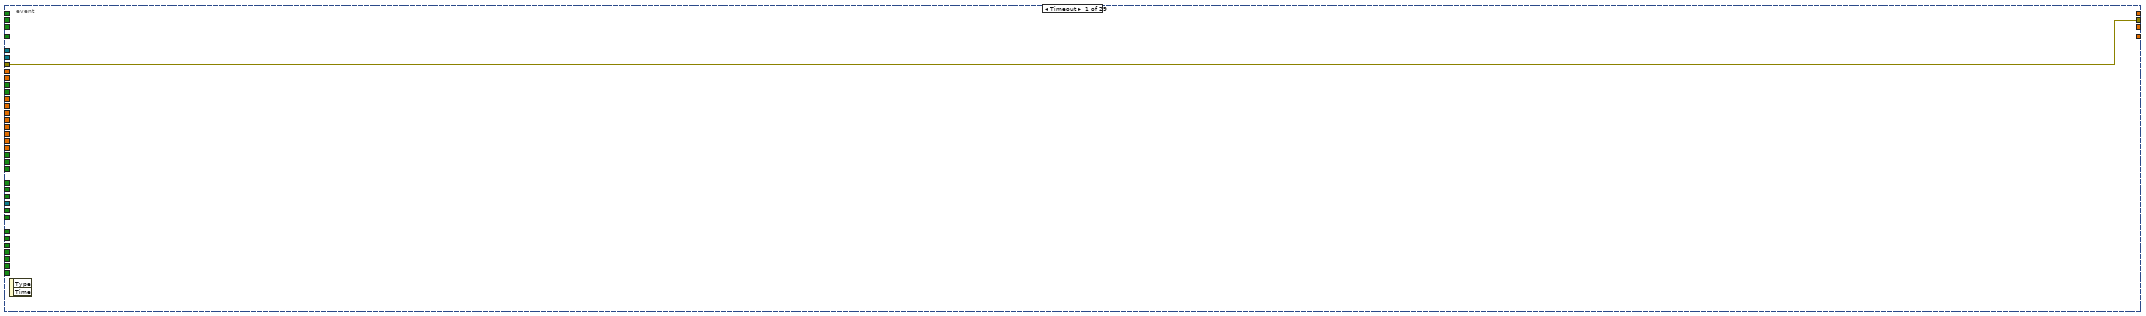
[diagram p7: hidden frame]
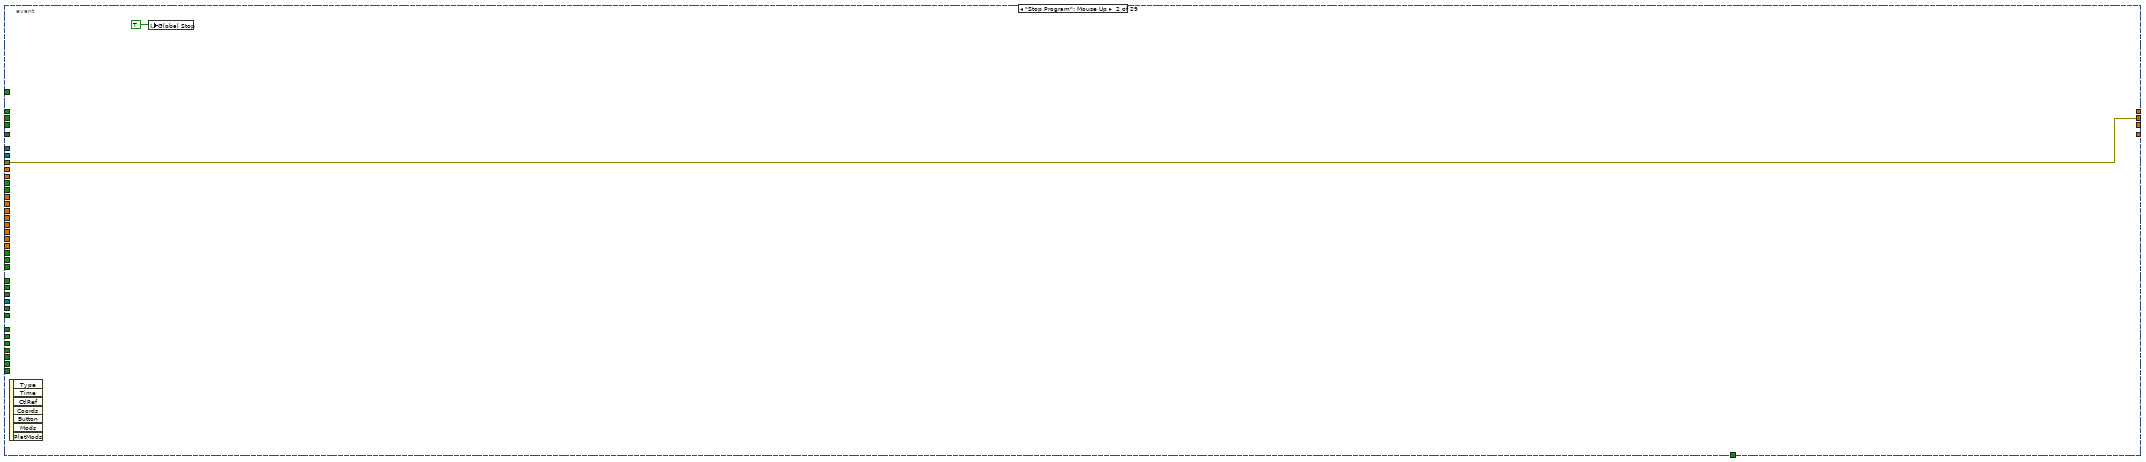
[diagram p8: hidden frame]
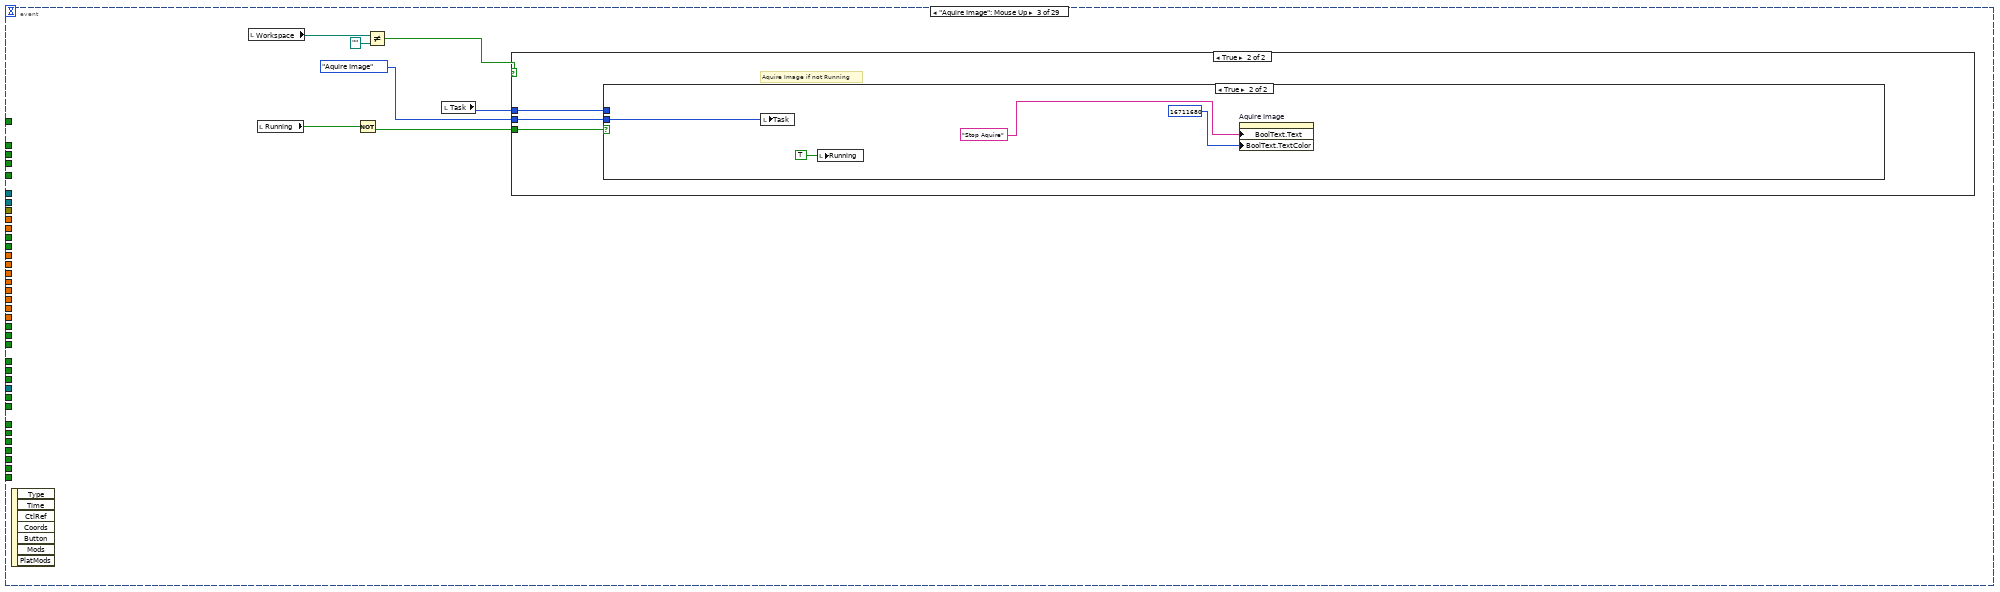
[diagram p9: hidden frame]
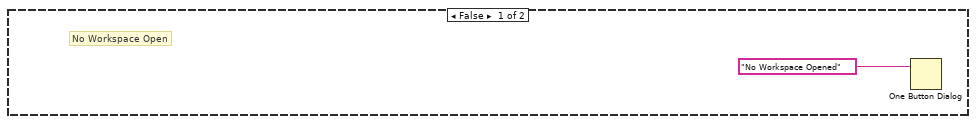
[diagram p10: hidden frame]
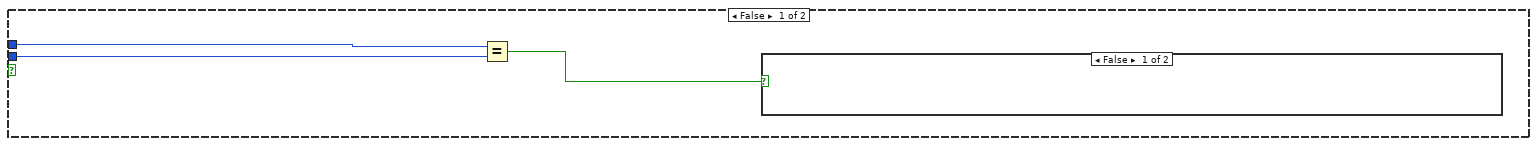
[diagram p11: hidden frame]
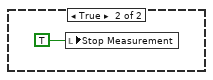
[diagram p12: hidden frame]
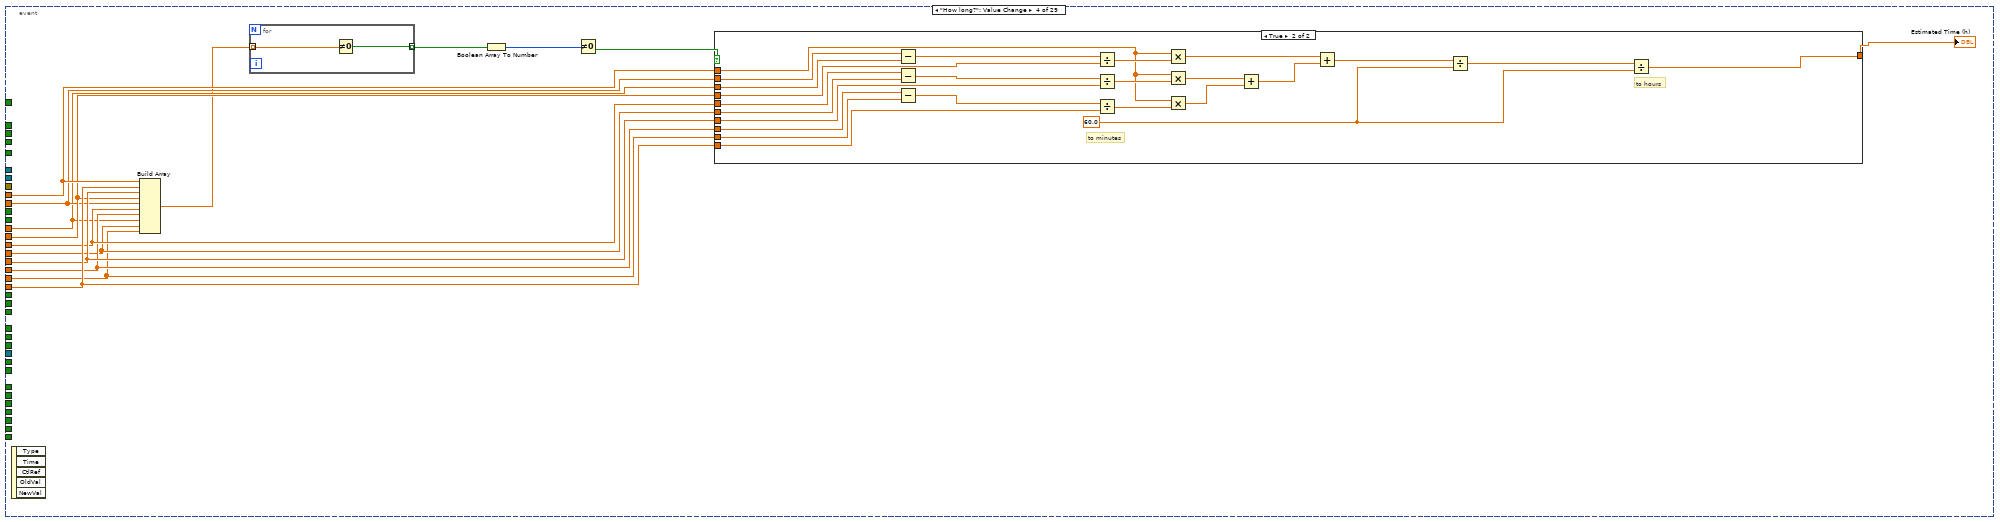
[diagram p13: hidden frame]
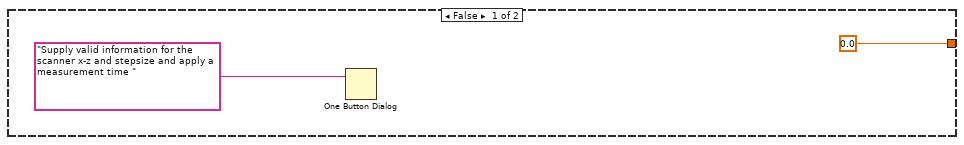
[diagram p14: hidden frame]
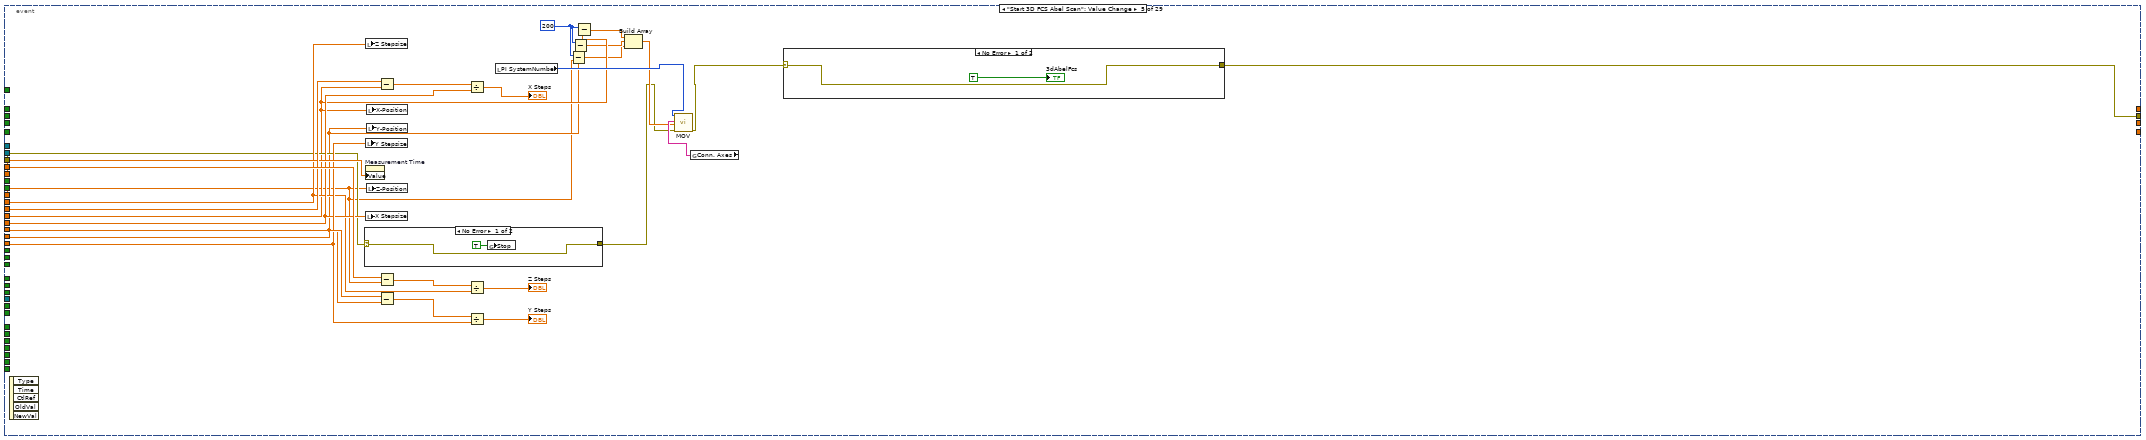
[diagram p15: hidden frame]
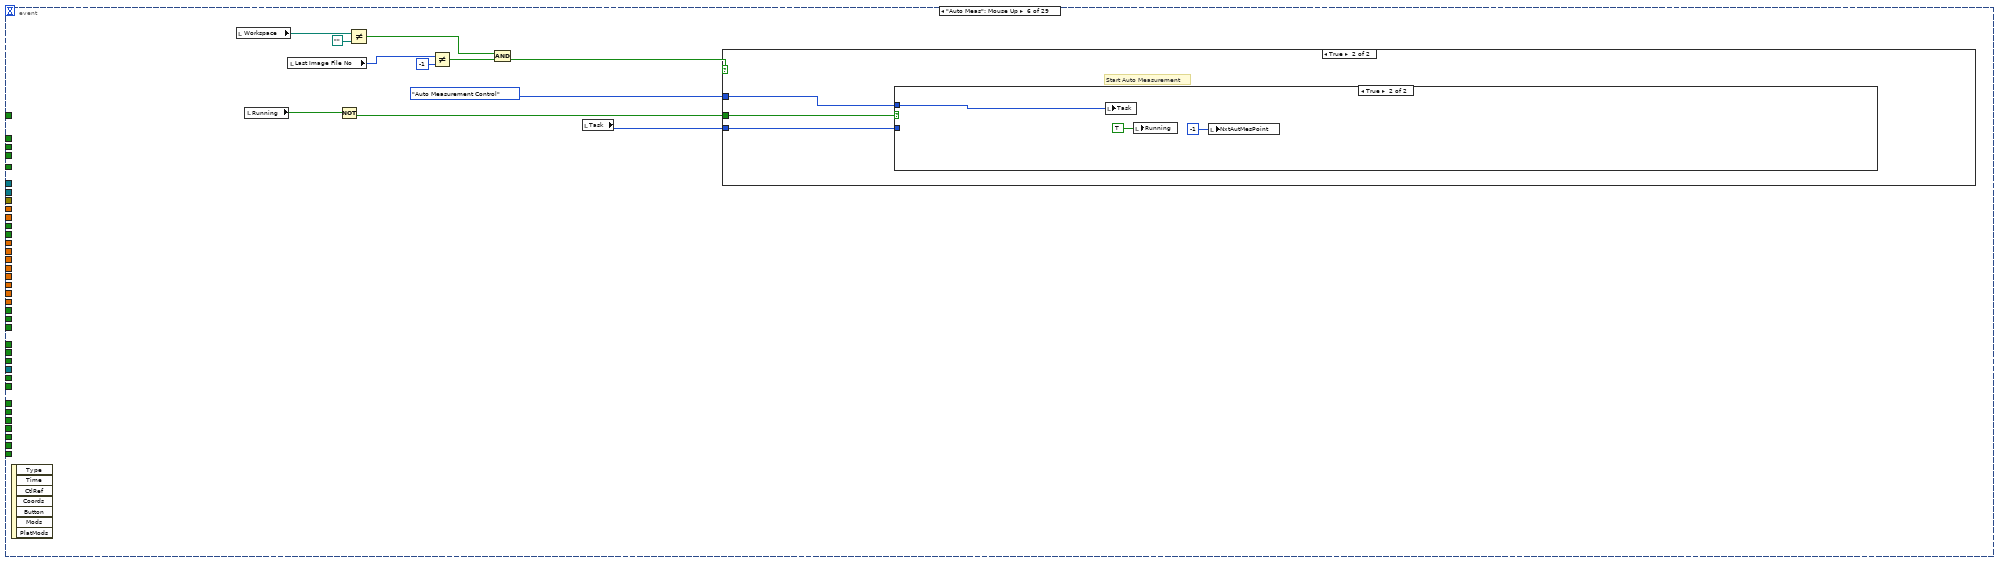
[diagram p18: hidden frame]
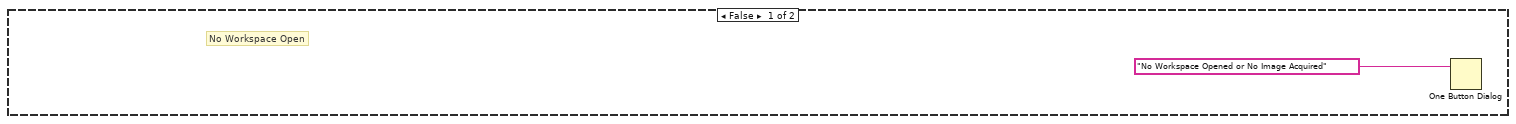
[diagram p19: hidden frame]
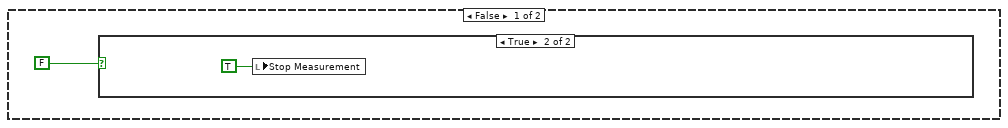
[diagram p20: hidden frame]
diagram:
  n1 = flat-sequence {
    tunnel: [w17] -> w11
    tunnel: errorcluster {"status"=FALSE, "code"=0, "source"=""} ("error in") -> [w28]
    frame #0 {
      (unwired) 1.0 ("CCD Chip Vertical Start")
      w29 = path ""
      w36 = FALSE ("Global Stop")
      n2 = control-ref of="WS File Tree"() -> (w35:refnum<vi>)
      n3 = global write "GetPicture.vi" "GetPicture"(FALSE ("GetPicture")) -> ()
      n4 = global write "GlobalSetGetConfigureCamera.vi" "gain"(30 ("gain")) -> ()
      n5 = local write "Last Image File No"(-1 ("Last Image File No")) -> ()
      n6 = global write "GlobalSetGetConfigureCamera.vi" "Exposure"(sgl 0.1 ("Exposure")) -> ()
      n7 = flat-sequence {
        tunnel: 1.0 ("Vertical Binning") -> [w42]
        tunnel: 1.0 ("CCD Chip Horizontal Start") -> [w41]
        tunnel: 1.0 ("CCD Chip Vertical Start") -> [w37]
        tunnel: 128.0 ("CCD Chip Horizontal End") -> [w40]
        tunnel: 128.0 ("CCD Chip Vertical End") -> [w39]
        tunnel: 1.0 ("Horizontal Binning") -> [w38]
        frame #0 {
          n8 = global write "GlobalSetGetConfigureCamera.vi" "Hbin"(w38) -> ()
          n9 = global write "GlobalSetGetConfigureCamera.vi" "Vbin"(w41) -> ()
          n10 = global write "GlobalSetGetConfigureCamera.vi" "Vbin"(w42) -> ()
          n11 = Subtract(x=w40, y=w41) -> (x-y=w44:dbl)
          n12 = Subtract(x=w39, y=w37) -> (x-y=w43:dbl)
          n13 = global write "ccdChipPixels.vi" "CCD Chip Vertical Start"(w37) -> ()
          n14 = global write "ccdChipPixels.vi" "CCD Chip horizontal start"(w37) -> ()
          n15 = global write "ccdChipPixels.vi" "CCD Chip Vertical end"(w39) -> ()
          n16 = global write "ccdChipPixels.vi" "CCD Chip horizontal end"(w40) -> ()
          n17 = Increment(x=w44) -> (x+1=w46:dbl)
          n18 = Increment(x=w43) -> (x+1=w45:dbl)
          n19 = Multiply(x=w46, y=w45) -> (x*y=w47:dbl)
          n20 = global write "ccdChipPixels.vi" "CCD Chip Size"(w47) -> ()
        }
      }
      n21 = property on="Aquire Image" class="Bool"("BoolText.Text"="Aquire Image" ("Caption.Text"), "BoolText.TextColor"=u32 0 ("Boolean Text.Colors:FG Color")) -> ()  [unwired: 2 in, 2 out]
      n22 = property on="Point Measurement" class="Bool"("BoolText.Text"="Point Measurement" ("Caption.Text"), "BoolText.TextColor"=u32 0 ("Boolean Text.Colors:FG Color")) -> ()  [unwired: 2 in, 2 out]
      n23 = local write "PI SystemNumber"(1 ("PI SystemNumber")) -> ()
      n24 = call "MTS_ClearWSTree2.vi"("error in"=w28, "Tree Refnum"=w35) -> ("error out"=w17:errorcluster)  [unwired: 8 in, 1 out]
      "Global Stop" <- w36
      "Running" <- w36
      "Buffer Overrun" <- w36
      "Stop Measurement" <- w36
      "Workspace" <- w29
      "Active pt3" <- w29
      "Task" <- T10."No Measurement" ("Do Measurement")
    }
  }
  n25 = local read "PI SystemNumber"() -> (w5:i32)
  n26 = control-ref of="X-Position"() -> (w10:refnum<vi>)
  n27 = control-ref of="Y-Position"() -> (w9:refnum<vi>)
  n28 = control-ref of="Z-Position"() -> (w8:refnum<vi>)
  n29 = call "AndorPhysikInstrumenteInitialisiation.vi"("reference"=w10, "error in (no error)"=w11, "reference 3"=w8, "reference 2"=w9, "Pi"=w5) -> ("error out"=w7:errorcluster, "Device List"=w15:T12)  [unwired: 5 in]
  n30 = case shown="True" FALSE {
    tunnel: w7 -> [_ w48]
    frame False {
    }
    frame True {
      n31 = while {
        tunnel: w48 -> [w49]
        tunnel: [w50] -> _
        stop <- w53 stop-if-true
        n32 = property on="3dAbelFcs" class="Bool (strict)"(error in=w49) -> (error out=w51:errorcluster, "Value"=w52:bool)  [unwired: 1 in, 1 out]
        n33 = local read "Global Stop"() -> (w53:bool)
        n34 = case shown="True" w52 {
          tunnel: w51 -> [_ w65]
          tunnel: [_ w71] -> w50
          frame False {
          }
          frame True {
            n35 = local read "Task"() -> (w58:T10)
            n36 = local read "Z Stepsize"() -> (w68:dbl)
            n37 = local read "Y Stepsize"() -> (w69:dbl)
            n38 = local read "X Stepsize"() -> (w70:dbl)
            n39 = local read "Z Steps"() -> (w67:dbl)
            n40 = Equal?(x=w58, y=T10."Auto Point" ("Task")) -> (x = y?=w56:bool)
            n41 = call "SetShutter.vi"("type"=Shutter_type_typedef."TTL High", "mode"=Shutter_mode_typedef."Open", "error in (no error)"=w65) -> ("error out"=w64:errorcluster)  [unwired: 11 in, 1 out]
            n42 = case shown="True" w56 {
              tunnel: w70 -> [w78 _]
              tunnel: w69 -> [w77 _]
              tunnel: w68 -> [w76 _]
              tunnel: w67 -> [w75 _]
              tunnel: [w74 w151] -> w66
              tunnel: w64 -> [w73 w162]
              tunnel: w56 -> [_ w163]
              frame False {
                n43 = for {
                  N: w75 -> [_]
                  tunnel: w73 -> [w87]
                  tunnel: w76 -> [w92]
                  tunnel: w77 -> [w91]
                  tunnel: w78 -> [w90]
                  tunnel: [w86] -> w74
                  tunnel: w75 -> [w85]
                  i -> [w89]
                  n44 = local read "Y Steps"() -> (w84:dbl)
                  n45 = local read "Z Start"() -> (w79:dbl)
                  n46 = Multiply(x=w92, y=w89) -> (x*y=w83:dbl)
                  n47 = Number To Decimal String(number=w89) -> (decimal integer string=w88:string)  [unwired: 1 in]
                  n48 = Subtract(x=200, y=w79) -> (x-y=w80:dbl)
                  n49 = Add(x=w80, y=w83) -> (x+y=w81:dbl)
                  n50 = for {
                    N: w84 -> [_]
                    tunnel: w91 -> [w130]
                    tunnel: w90 -> [w129]
                    tunnel: w87 -> [w126]
                    tunnel: w88 -> [w128]
                    tunnel: [w100] -> w86
                    tunnel: w79 -> [w97]
                    tunnel: w85 -> [w121]
                    tunnel: w84 -> [w120]
                    tunnel: w81 -> [w118]
                    i -> [w102]
                    w98 = "_" ("string")
                    n51 = Multiply(x=w130, y=w102) -> (x*y=w125:dbl)
                    n52 = Increment(x=w102) -> (x+1=w103:i32)
                    n53 = local read "X Steps"() -> (w119:dbl)
                    n54 = local read "Y Start"() -> (w93:dbl)
                    n55 = Number To Decimal String(number=w102) -> (decimal integer string=w127:string)  [unwired: 1 in]
                    n56 = property on="Workspace" class="Path"() -> ("Value"=w99:path)  [unwired: 2 in, 2 out]
                    n57 = Number To Decimal String(number=w103) -> (decimal integer string=w109:string)  [unwired: 1 in]
                    n58 = for {
                      N: w119 -> [_]
                      tunnel: w126 -> [w145]
                      tunnel: w129 -> [w150]
                      tunnel: [w146] -> w124
                      tunnel: w128 -> [w148]
                      tunnel: w127 -> [w147]
                      shift-right: [w144] -> w123
                      shift-left: _ -> [w143]
                      tunnel: [w142] -> w122
                      tunnel: [w140] -> w117
                      tunnel: [w141] -> w116
                      i -> [w149]
                      n59 = control-ref of="Running"() -> (w139:refnum<vi>)
                      n60 = control-ref of="Workspace"() -> (w137:refnum<vi>)
                      n61 = control-ref of="FCS Point Measurement"() -> (w134:refnum<vi>)
                      n62 = control-ref of="Stop Measurement"() -> (w136:refnum<vi>)
                      n63 = control-ref of="Point Measurement"() -> (w131:refnum<vi>)
                      n64 = control-ref of="concatenated string"() -> (w132:refnum<vi>)
                      n65 = control-ref of="X-Position"() -> (w135:refnum<vi>)
                      n66 = control-ref of="X Start"() -> (w133:refnum<vi>)
                      n67 = control-ref of="Task"() -> (w138:refnum<vi>)
                      n68 = call "LifeTimeImagePoint.vi"("Boolean in"=w139, "String"=w147, "reference 6"=w135, "String 2"=w148, "reference 7"=w134, "error in (no error)"=w145, "reference 4"=w136, "reference 3"=w137, "reference 9"=w133, "reference in"=w138, "Numeric in"=w149, "Str Refnum"=w132, "X Stepsize"=w150, "Array in"=w143, "Point Measurement"=w131) -> ("Array out"=w144:i32[][], "CCD Chip Size"=w141:i32, "X Start"=w142:dbl, "Numeric out"=w140:dbl, "error out"=w146:errorcluster)  [unwired: 8 in]
                    }
                    n69 = Strip Path(path=w99) -> (stripped path=w112:path)  [unwired: 1 out]
                    n70 = Subtract(x=200, y=w93) -> (x-y=w94:dbl)
                    n71 = Add(x=w94, y=w125) -> (x+y=w95:dbl)
                    n72 = Path To String(path=w112) -> (string=w113:string)
                    n73 = Get Date/Time In Seconds() -> (seconds since 1Jan1904=w108:timestamp)
                    n74 = local write "Y-Position"(w93) -> ()
                    n75 = Format Date/Time String(time format string (%c)="%d%m%y_%H%M", seconds (now)=w108) -> (date/time string=w106:string)  [unwired: 1 in]
                    n76 = Concatenate Strings(w113, "\\" ("string"), "AreaISM" ("string"), w98, w109, w98, w106, w98, w98) -> (w114:string)
                    n77 = String To Path(string=w114) -> (path=w105:path)
                    n78 = Path To String(path=w105) -> (string=w104:string)
                    n79 = Build Array(w97, w93, w122, w121, w120, w119, w118, w95, w117, w116) -> (w115:dbl[])
                    n80 = script code="results.ImagePlane=Data;\nresults.Info.Zstart=Meta(1);\nresults.Info.Ystart=Meta(2);\nresults.Info.Xstart=Meta(3);\nresults.Info.Zsteps=Meta(4);\nresults.Info.Ysteps=Meta(5);\nresults.Info.Xsteps=Meta(6);\nresults.Info.Zpos=Meta(7);\nresults.Info.Ypos=Meta(8);\nresults.Info.Xpos=Meta(9);\nresults.Info.CcdSize=Meta(13);\nsave(file,'results');\nclear results;"("??"=w124, "Data"=w123, "Meta"=w115, "file"=w104) -> ("??"=w101:errorcluster)
                    n81 = call "FreeInternalMemory.vi"("error in (no error)"=w101) -> ("error out"=w100:errorcluster)  [unwired: 1 in, 1 out]
                  }
                  n82 = local write "Z-Position"(w79) -> ()
                }
              }
              frame True {
                w169 = "_" ("string")
                n83 = call "StartAcquisition.vi"("error in (no error)"=w161) -> ("error out"=w180:errorcluster)  [unwired: 1 in, 1 out]
                n84 = flat-sequence {
                  tunnel: w163 -> [w199]
                  tunnel: w162 -> [w194]
                  tunnel: [w194] -> w161
                  tunnel: [w183] -> w160
                  tunnel: [w182] -> w159
                  tunnel: [w181] -> w158
                  frame #0 {
                    w187 = 200
                    n85 = local read "x-position"() -> (w193:dbl)
                    n86 = local read "y-position"() -> (w192:dbl)
                    n87 = local read "z-position"() -> (w191:dbl)
                    n88 = local read "NxtAutMesPoint"() -> (w198:i32)
                    n89 = Subtract(x=w187, y=w191) -> (x-y=w188:dbl)
                    n90 = Subtract(x=w187, y=w192) -> (x-y=w189:dbl)
                    n91 = Subtract(x=w187, y=w193) -> (x-y=w190:dbl)
                    n92 = local read "Pattern"() -> (w197:dbl[][])
                    n93 = Bundle(w190, w189, w188) -> (w196:cluster{dbl, dbl, dbl})  [unwired: 1 in]
                    n94 = call "MTS_AutoPointCords.vi"("Is Auto Point"=w199, "Cords In"=w196, "Next Auto Measure Point"=w198, "Pattern"=w197) -> ("Cords"=w195:T16)  [unwired: 7 in]
                    n95 = Unbundle By Name(w195) -> ("X-Position"=w186:dbl, "Y-Position"=w185:dbl, "Z-Position"=w184:dbl)
                    n96 = Subtract(x=w187, y=w184) -> (x-y=w181:dbl)
                    n97 = Subtract(x=w187, y=w185) -> (x-y=w182:dbl)
                    n98 = Subtract(x=w187, y=w186) -> (x-y=w183:dbl)
                  }
                }
                n99 = while {
                  tunnel: w180 -> [w200]
                  tunnel: [w203] -> w178
                  stop <- w202 stop-if-true
                  n100 = call "GetStatus.vi"("error in (no error)"=w200) -> ("error out"=w203:errorcluster, "status"=w204:T15)  [unwired: 2 in, 1 out]
                  n101 = Wait (ms)(milliseconds to wait=u32 100) -> ()  [unwired: 1 out]
                  n102 = Equal?(x=Error_Code_Enum_typedef."DRV_IDLE" ("status"), y=w204) -> (x = y?=w202:bool)
                }
                n103 = global read "ccdChipPixels.vi" "CCD Chip Size"() -> (w155:i32)
                n104 = call "GetAcquiredData.vi"("error in (no error)"=w178, "size"=w155) -> ("error out"=w179:errorcluster, "array"=w164:i32[])  [unwired: 1 in, 1 out]
                n105 = call <vilib>:"Clear Errors.vi"("error in (no error)"=w179) -> ("error out"=w153:errorcluster)  [unwired: 6 in]
                n106 = local read "NxtAutMesPoint"() -> (w157:i32)
                n107 = property on="Workspace" class="Path"() -> ("Value"=w168:path)  [unwired: 2 in, 2 out]
                n108 = Number To Decimal String(number=w157) -> (decimal integer string=w173:string)  [unwired: 1 in]
                n109 = Strip Path(path=w168) -> (stripped path=w176:path)  [unwired: 1 out]
                n110 = Path To String(path=w176) -> (string=w177:string)
                n111 = Get Date/Time In Seconds() -> (seconds since 1Jan1904=w172:timestamp)
                n112 = Format Date/Time String(time format string (%c)="%d%m%y_%H%M", seconds (now)=w172) -> (date/time string=w170:string)  [unwired: 1 in]
                n113 = global read "GlobalSetGetConfigureCamera.vi" "Exposure"() -> (w156:sgl)
                n114 = Concatenate Strings(w177, "\\" ("string"), "DefocussedPointMes" ("string"), w169, w173, w169, w170, w169, w169) -> (w166:string)
                n115 = Build Array(w160, w159, w158, w157, w156, w155) -> (w154:dbl[])
                n116 = String To Path(string=w166) -> (path=w167:path)
                n117 = Path To String(path=w167) -> (string=w165:string)
                n118 = script code="results.ImagePlane=Data;\nresults.Info.PositionX=Meta(1);\nresults.Info.PositionY=Meta(2);\nresults.Info.PositionZ=Meta(3);\nresults.Info.AutoMesPoint=Meta(4);\nresults.Info.Ex=Meta(5);\nresults.Info.CcdSize=Meta(13);\nsave(file,'results');\nclear results;"("??"=w153, "Data"=w164, "Meta"=w154, "file"=w165) -> ("??"=w152:errorcluster)
                n119 = call <vilib>:"Clear Errors.vi"("error in (no error)"=w152) -> ("error out"=w151:errorcluster)  [unwired: 6 in]
              }
            }
            n120 = call "AbortAcquisition.vi"("error in (no error)"=w66) -> ("error out"=w62:errorcluster)  [unwired: 1 in, 1 out]
            n121 = call "SetShutter.vi"("type"=Shutter_type_typedef."TTL High", "mode"=Shutter_mode_typedef."Close", "error in (no error)"=w62) -> ("error out"=w55:errorcluster)  [unwired: 11 in, 1 out]
            n122 = call <vilib>:"Clear Errors.vi"("error in (no error)"=w55) -> ("error out"=w54:errorcluster)  [unwired: 6 in]
            n123 = property on="3dAbelFcs" class="Bool (strict)"(error in=w54, "Value"=FALSE ("3dAbelFcs")) -> (error out=w71:errorcluster)  [unwired: 1 in, 1 out]
          }
        }
      }
    }
  }
  n124 = while {
    shift-right: [w244] -> _
    shift-left: w7 -> [w246]
    stop <- w245 stop-if-true
    n125 = local read "Global Stop"() -> (w245:bool)
    n126 = control-ref of="WS File Tree"() -> (w219:refnum<vi>)
    n127 = global read "GlobalLaserInterface.vi" "InterfaceLaserInitalised"() -> (w207:refnum<visa-resource-name>)
    n128 = event shown="[17] \"SCANNER EMERGENCY\": Value Change" {
      selector: _ -> [_ _ _ _ _ _ _ _ _ _ _ _ _ _ _ _ _ _ _ _ _ _ _ _ _ _ _ _ _]
      dyn-events: _ -> [_ _ _ _ _ _ _ _ _ _ _ _ _ _ _ _ _ _ _ _ _ _ _ _ _ _ _ _ _]
      timeout: _ -> [_ _ _ _ _ _ _ _ _ _ _ _ _ _ _ _ _ _ _ _ _ _ _ _ _ _ _ _ _]
      tunnel: w246 -> [w247 w249 _ _ w324 _ w367 _ _ _ w410 w463 w466 w502 _ w562 _ w602 w609 w638 _ w648 w657 w668 w670 _ _ _ w677]
      tunnel: [w247 w249 _ _ w325 _ w366 _ _ _ w409 w455 w464 w499 _ w561 _ w601 _ _ _ w646 _ w667 _ _ _ _ w678] -> w244
      tunnel: w219 -> [_ _ _ _ _ _ _ _ _ _ _ _ w468 w503 _ _ _ _ _ _ _ _ _ _ _ _ _ _ _]
      tunnel: "Aquire Image" -> [_ _ _ _ _ _ _ _ _ _ _ _ _ _ _ _ _ _ _ _ _ _ _ _ _ _ _ _ _]
      tunnel: "Save Color Image" -> [_ _ _ _ _ _ _ _ _ _ _ _ _ _ _ _ _ _ _ _ _ _ _ _ _ _ _ _ _]
      tunnel: "Open MSW" -> [_ _ _ _ _ _ _ _ _ _ _ _ _ _ _ _ _ _ _ _ _ _ _ _ _ _ _ _ _]
      tunnel: "Find Mols" -> [_ _ _ _ _ _ _ _ _ _ _ _ _ _ _ _ _ _ _ _ _ _ _ _ _ _ _ _ _]
      tunnel: "Auto Meas" -> [_ _ _ _ _ _ _ _ _ _ _ _ _ _ _ _ _ _ _ _ _ _ _ _ _ _ _ _ _]
      tunnel: "New MSW" -> [_ _ _ _ _ _ _ _ _ _ _ _ _ _ _ _ _ _ _ _ _ _ _ _ _ _ _ _ _]
      tunnel: "Stop Program" -> [_ _ _ _ _ _ _ _ _ _ _ _ _ _ _ _ _ _ _ _ _ _ _ _ _ _ _ _ _]
      tunnel: "Point Measurement" -> [_ _ _ _ _ _ _ _ _ _ _ _ _ _ _ _ _ _ _ _ _ _ _ _ _ _ _ _ _]
      tunnel: "Move Stage" -> [_ _ _ _ _ _ _ _ _ _ _ _ _ _ _ _ _ _ _ _ _ _ _ _ _ _ _ _ _]
      tunnel: w207 -> [_ _ _ _ _ _ _ _ _ _ _ _ _ _ _ _ _ _ _ _ _ _ _ _ _ _ _ _ _]
      tunnel: "Get Position" -> [_ _ _ _ _ _ _ _ _ _ _ _ _ _ _ _ _ _ _ _ _ _ _ _ _ _ _ _ _]
      tunnel: [_ _ _ _ _ _ _ _ _ _ w405 w448 _ _ _ _ _ _ _ _ _ _ _ _ _ _ _ _ _] -> w234
      tunnel: [_ _ _ _ _ _ _ _ _ _ w406 w449 _ _ _ _ _ _ _ _ _ _ _ _ _ _ _ _ _] -> w218
      tunnel: [_ _ _ _ _ _ _ _ _ _ w407 w450 _ _ _ _ _ _ _ _ _ _ _ _ _ _ _ _ _] -> w233
      tunnel: "How long?" -> [_ _ _ _ _ _ _ _ _ _ _ _ _ _ _ _ _ _ _ _ _ _ _ _ _ _ _ _ _]
      tunnel: "Start 3D FCS Abel Scan" -> [_ _ _ _ _ _ _ _ _ _ _ _ _ _ _ _ _ _ _ _ _ _ _ _ _ _ _ _ _]
      tunnel: "Mesaurement Time (Sec) / Step" -> [_ _ _ w283 w329 _ _ _ _ _ _ _ _ _ _ _ _ _ _ _ _ _ _ _ _ _ w675 _ _]
      tunnel: "Y Stepsize" -> [_ _ _ w282 w328 _ _ _ _ _ _ _ _ _ _ _ _ _ _ _ _ _ _ _ _ _ _ _ _]
      tunnel: "X Stepsize" -> [_ _ _ w281 w327 _ _ _ _ _ _ _ _ _ _ _ _ _ _ _ _ _ _ _ _ _ _ _ _]
      tunnel: "Z Stepsize" -> [_ _ _ w280 w326 _ _ _ _ _ _ _ _ _ _ _ _ _ _ _ _ _ _ _ _ _ _ _ _]
      tunnel: "FCS Point Measurement" -> [_ _ _ _ _ _ _ _ _ _ _ _ _ _ _ _ _ _ _ _ _ _ _ _ _ _ _ _ _]
      tunnel: "Z End" -> [_ _ _ w279 w338 _ _ _ _ _ _ _ _ _ _ _ _ _ _ _ _ _ _ _ _ _ _ _ _]
      tunnel: "X End" -> [_ _ _ w278 w332 _ _ _ _ _ _ _ _ _ _ _ _ _ _ _ _ _ _ _ _ _ _ _ _]
      tunnel: "Y End" -> [_ _ _ w277 w335 _ _ _ _ _ _ _ _ _ _ _ _ _ _ _ _ _ _ _ _ _ _ _ _]
      tunnel: "Z Start" -> [_ _ _ w276 w318 _ _ _ _ _ _ _ _ _ _ _ _ _ _ _ _ _ _ _ _ _ _ _ _]
      tunnel: "X Start" -> [_ _ _ w275 w320 _ _ _ _ _ _ _ _ _ _ _ _ _ _ _ _ _ _ _ _ _ _ _ _]
      tunnel: "Y Start" -> [_ _ _ w274 w319 _ _ _ _ _ _ _ _ _ _ _ _ _ _ _ _ _ _ _ _ _ _ _ _]
      tunnel: w219 -> [_ _ _ _ _ _ _ _ _ _ _ _ _ _ _ _ _ _ _ _ _ _ _ _ _ _ _ _ _]
      tunnel: "SET CCD" -> [_ _ _ _ _ _ _ _ _ _ _ _ _ _ _ _ _ _ _ _ _ _ _ _ _ _ _ _ _]
      tunnel: "OPEN SHUTER" -> [_ _ _ _ _ _ _ _ _ _ _ _ _ _ _ _ _ _ _ _ _ w647 _ _ _ _ _ _ _]
      tunnel: "Close" -> [_ _ _ _ _ _ _ _ _ _ _ _ _ _ _ _ _ _ _ _ _ _ w656 _ _ _ _ _ _]
      tunnel: "Stop" -> [_ _ _ _ _ _ _ _ _ _ _ _ _ _ _ _ _ _ _ _ _ _ _ _ _ _ _ _ _]
      tunnel: "Start" -> [_ _ _ _ _ _ _ _ _ _ _ _ _ _ _ _ _ _ _ _ _ _ _ _ _ _ _ _ _]
      tunnel: "Gain" -> [_ _ _ _ _ _ _ _ _ _ _ _ _ _ _ _ _ _ _ _ _ _ _ _ _ _ _ _ _]
      tunnel: "Cam (Defocused)" -> [_ _ _ _ _ _ _ _ _ _ _ _ _ _ _ _ _ _ _ _ w645 _ _ _ _ _ _ _ _]
      tunnel: "Set Temperature" -> [_ _ _ _ _ _ _ _ _ _ _ _ _ _ _ _ _ _ _ _ _ _ _ _ _ _ _ _ _]
      tunnel: "SCANNER EMERGENCY" -> [_ _ _ _ _ _ _ _ _ _ _ _ _ _ _ _ _ _ _ _ _ _ _ _ _ _ _ _ _]
      tunnel: "Get Temperature" -> [_ _ _ _ _ _ _ _ _ _ _ _ _ _ _ _ _ _ _ _ _ _ _ _ _ _ _ _ _]
      event Timeout {
        n129 = event-data() -> ()  [unwired: 1 in, 2 out]
      }
      event "Stop Program": Mouse Up {
        n130 = event-data() -> ()  [unwired: 1 in, 7 out]
        n131 = local write "Global Stop"(TRUE ("Global Stop")) -> ()
      }
      event "Aquire Image": Mouse Up {
        n132 = event-data() -> ()  [unwired: 1 in, 7 out]
        n133 = local read "Workspace"() -> (w253:path)
        n134 = local read "Running"() -> (w256:bool)
        n135 = Not(x=w256) -> (.not. x?=w255:bool)
        n136 = Not Equal?(x=w253, y=path "") -> (x != y?=w251:bool)
        n137 = local read "Task"() -> (w250:T10)
        n138 = case shown="True" w251 {
          tunnel: w255 -> [_ w260]
          tunnel: T17."Aquire Image" ("Do Measurement") -> [_ w259]
          tunnel: w250 -> [_ w258]
          frame False {
            # "No Workspace Open"
            n139 = One Button Dialog(message="No Workspace Opened") -> ()  [unwired: 1 in, 1 out]
          }
          frame True {
            # "Aquire Image if not Running"
            n140 = case shown="True" w260 {
              tunnel: w259 -> [w263 w266]
              tunnel: w258 -> [w261 _]
              frame False {
                n141 = Equal?(x=w261, y=w263) -> (x = y?=w262:bool)
                n142 = case shown="False" w262 {
                  frame False {
                  }
                  frame True {
                    n143 = local write "Stop Measurement"(TRUE ("Stop Measurement")) -> ()
                  }
                }
              }
              frame True {
                n144 = local write "Task"(w266) -> ()
                n145 = local write "Running"(TRUE ("Measurement Running")) -> ()
                n146 = property on="Aquire Image" class="Bool"("BoolText.Text"="Stop Aquire" ("Caption.Text"), "BoolText.TextColor"=u32 16711680 ("Boolean Text.Colors:FG Color")) -> ()  [unwired: 2 in, 2 out]
              }
            }
          }
        }
      }
      event "How long?": Value Change {
        n147 = event-data() -> ()  [unwired: 1 in, 5 out]
        n148 = Build Array(w283, w282, w281, w280, w279, w278, w277, w276, w275, w274) -> (w273:dbl[])
        n149 = for {
          tunnel: w273 -> [w311] mode=indexing
          tunnel: [w310] -> w272 mode=indexing
          n150 = Not Equal To 0?(x=w311) -> (x != 0?=w310:bool)
        }
        n151 = Boolean Array To Number(Boolean array=w272) -> (number=w271:u32)
        n152 = Not Equal To 0?(x=w271) -> (x != 0?=w270:bool)
        n153 = case shown="True" w270 {
          tunnel: [0.0 w296] -> w269
          tunnel: w283 -> [_ w295]
          tunnel: w282 -> [_ w294]
          tunnel: w281 -> [_ w293]
          tunnel: w280 -> [_ w292]
          tunnel: w279 -> [_ w291]
          tunnel: w278 -> [_ w290]
          tunnel: w277 -> [_ w289]
          tunnel: w276 -> [_ w288]
          tunnel: w275 -> [_ w287]
          tunnel: w274 -> [_ w286]
          frame False {
            n154 = One Button Dialog(message="Supply valid information for the scanner x-z and stepsize and apply a measurement time ") -> ()  [unwired: 1 in, 1 out]
          }
          frame True {
            w297 = 60.0 ("y")
            # "to hours"
            # "to minutes"
            n155 = Subtract(x=w291, y=w288) -> (x-y=w304:dbl)
            n156 = Subtract(x=w290, y=w287) -> (x-y=w309:dbl)
            n157 = Subtract(x=w289, y=w286) -> (x-y=w306:dbl)
            n158 = Divide(x=w304, y=w292) -> (x/y=w305:dbl)
            n159 = Divide(x=w309, y=w293) -> (x/y=w308:dbl)
            n160 = Divide(x=w306, y=w294) -> (x/y=w307:dbl)
            n161 = Multiply(x=w295, y=w305) -> (x*y=w301:dbl)
            n162 = Multiply(x=w295, y=w308) -> (x*y=w303:dbl)
            n163 = Multiply(x=w295, y=w307) -> (x*y=w302:dbl)
            n164 = Add(x=w303, y=w302) -> (x+y=w300:dbl)
            n165 = Add(x=w301, y=w300) -> (x+y=w299:dbl)
            n166 = Divide(x=w299, y=w297) -> (x/y=w298:dbl)
            n167 = Divide(x=w298, y=w297) -> (x/y=w296:dbl)
          }
        }
        "Estimated Time (h)" <- w269
      }
      event "Start 3D FCS Abel Scan": Value Change {
        w321 = 200
        n168 = event-data() -> ()  [unwired: 1 in, 5 out]
        n169 = case shown="No Error" w324 {
          selector: w324 -> [w339 w341]
          tunnel: [w339 w341] -> w313
          frame No Error {
            n170 = global write "StopGetPic.vi" "Stop"(TRUE ("Stop")) -> ()
          }
          frame Error {
          }
        }
        n171 = local write "Z Stepsize"(w326) -> ()
        n172 = local write "Y Stepsize"(w328) -> ()
        n173 = property on="Measurement Time" class="DigNum (strict)"("Value"=w329) -> ()  [unwired: 2 in, 2 out]
        n174 = local write "X Stepsize"(w327) -> ()
        n175 = local write "X-Position"(w320) -> ()
        n176 = local write "Y-Position"(w319) -> ()
        n177 = local write "Z-Position"(w318) -> ()
        n178 = Subtract(x=w332, y=w320) -> (x-y=w331:dbl)
        n179 = Subtract(x=w338, y=w318) -> (x-y=w336:dbl)
        n180 = Subtract(x=w335, y=w319) -> (x-y=w334:dbl)
        n181 = Divide(x=w331, y=w327) -> (x/y=→"X Steps":dbl)
        n182 = Divide(x=w336, y=w326) -> (x/y=→"Z Steps":dbl)
        n183 = Divide(x=w334, y=w328) -> (x/y=→"Y Steps":dbl)
        n184 = local read "PI SystemNumber"() -> (w323:i32)
        n185 = Subtract(x=w321, y=w318) -> (x-y=w315:dbl)
        n186 = Subtract(x=w321, y=w319) -> (x-y=w316:dbl)
        n187 = Subtract(x=w321, y=w320) -> (x-y=w317:dbl)
        n188 = Build Array(w317, w316, w315) -> (w314:dbl[])
        n189 = global read "GlobalConAxisPI.vi" "Conn. Axes"() -> (w322:string[])
        n190 = call "MOV.vi"("System no."=w323, "Axes to move"=w322, "Position values"=w314, "error in"=w313) -> ("error out"=w312:errorcluster)  [unwired: 15 in]
        n191 = case shown="No Error" w312 {
          selector: w312 -> [w342 w344]
          tunnel: [w342 w344] -> w325
          frame No Error {
            "3dAbelFcs" <- TRUE
          }
          frame Error {
          }
        }
      }
      event "Auto Meas": Mouse Up {
        n192 = event-data() -> ()  [unwired: 1 in, 7 out]
        n193 = local read "Workspace"() -> (w352:path)
        n194 = local read "Running"() -> (w355:bool)
        n195 = local read "Last Image File No"() -> (w349:i32)
        n196 = Not(x=w355) -> (.not. x?=w354:bool)
        n197 = Not Equal?(x=w352, y=path "") -> (x != y?=w347:bool)
        n198 = Not Equal?(x=w349, y=-1) -> (x != y?=w346:bool)
        n199 = And(x=w347, y=w346) -> (x .and. y?=w345:bool)
        n200 = local read "Task"() -> (w353:T10)
        n201 = case shown="True" w345 {
          tunnel: w354 -> [_ w359]
          tunnel: T18."Auto Measurement Control" ("Do Measurement") -> [_ w358]
          tunnel: w353 -> [_ w357]
          frame False {
            # "No Workspace Open"
            n202 = One Button Dialog(message="No Workspace Opened or No Image Acquired") -> ()  [unwired: 1 in, 1 out]
          }
          frame True {
            # "Start Auto Measurement"
            n203 = case shown="True" w359 {
              tunnel: w358 -> [_ w363]
              tunnel: w357 -> [_ _]
              frame False {
                n204 = case shown="True" FALSE {
                  frame False {
                  }
                  frame True {
                    n205 = local write "Stop Measurement"(TRUE ("Stop Measurement")) -> ()
                  }
                }
              }
              frame True {
                n206 = local write "Task"(w363) -> ()
                n207 = local write "Running"(TRUE ("Measurement Running")) -> ()
                n208 = local write "NxtAutMesPoint"(-1 ("NxtAutMesPoint")) -> ()
              }
            }
          }
        }
      }
      event "Get Temperature": Value Change {
        n209 = event-data() -> ()  [unwired: 1 in, 5 out]
        n210 = call "GetTemperature.vi"("error in (no error)"=w367) -> ("error out"=w368:errorcluster, "temperature"=w371:i32)  [unwired: 3 in, 2 out]
        n211 = call "Build Text"("Cam"=w371, "error in (no error)"=w368) -> ("Result"=w370:string, "error out"=w369:errorcluster)  [unwired: 12 in]
        n212 = call "Display Message to User"("error in (no error)"=w369, "Enable"=TRUE, "Message"=w370) -> ("error out"=w366:errorcluster)  [unwired: 7 in, 1 out]
      }
      event "Save Color Image": Mouse Up {
        n213 = event-data() -> ()  [unwired: 1 in, 7 out]
        n214 = local read "Active pt3"() -> (w374:path)
        n215 = Not Equal?(x=w374, y=path "") -> (x != y?=w372:bool)
        n216 = case shown="True" w372 {
          tunnel: T19."Save Color Image" ("Do Measurement") -> [_ w378]
          frame False {
            # "No Workspace Open"
            n217 = One Button Dialog(message="No pt3 File opened") -> ()  [unwired: 1 in, 1 out]
          }
          frame True {
            # "Aquire Image if not Running"
            n218 = local write "Task"(w378) -> ()
            n219 = local write "Running"(TRUE ("Measurement Running")) -> ()
          }
        }
      }
      event "Find Mols": Mouse Up {
        n220 = event-data() -> ()  [unwired: 1 in, 7 out]
        n221 = local read "Active pt3"() -> (w381:path)
        n222 = Not Equal?(x=w381, y=path "") -> (x != y?=w379:bool)
        n223 = case shown="True" w379 {
          tunnel: T19."Find Single Mol." ("Do Measurement") -> [_ w385]
          frame False {
            # "No Workspace Open"
            n224 = One Button Dialog(message="No pt3 File opened") -> ()  [unwired: 1 in, 1 out]
          }
          frame True {
            # "Aquire Image if not Running"
            n225 = local write "Task"(w385) -> ()
            n226 = local write "Running"(TRUE ("Measurement Running")) -> ()
          }
        }
      }
      event "Point Measurement": Mouse Up {
        n227 = event-data() -> ()  [unwired: 1 in, 7 out]
        n228 = local read "Workspace"() -> (w388:path)
        n229 = local read "Running"() -> (w392:bool)
        n230 = Not(x=w392) -> (.not. x?=w391:bool)
        n231 = Not Equal?(x=w388, y=path "") -> (x != y?=w386:bool)
        n232 = local read "Task"() -> (w389:T10)
        n233 = case shown="True" w386 {
          tunnel: w391 -> [_ w396]
          tunnel: T17."Point Measurement" ("Do Measurement") -> [_ w395]
          tunnel: w389 -> [_ w394]
          frame False {
            # "No Workspace Open"
            n234 = One Button Dialog(message="No Workspace Opened") -> ()  [unwired: 1 in, 1 out]
          }
          frame True {
            # "Aquire Image if not Running"
            n235 = case shown="False" w396 {
              tunnel: w395 -> [w398 w402]
              tunnel: w394 -> [w399 _]
              frame False {
                n236 = Equal?(x=w399, y=w398) -> (x = y?=w397:bool)
                n237 = case shown="False" w397 {
                  frame False {
                  }
                  frame True {
                    n238 = local write "Stop Measurement"(TRUE ("Stop Measurement")) -> ()
                  }
                }
              }
              frame True {
                n239 = local write "Task"(w402) -> ()
                n240 = local write "Running"(TRUE ("Measurement Running")) -> ()
                n241 = property on="Point Measurement" class="Bool"("BoolText.Text"="Stop Aquire" ("Caption.Text"), "BoolText.TextColor"=u32 16711680 ("Boolean Text.Colors:FG Color")) -> ()  [unwired: 2 in, 2 out]
              }
            }
          }
        }
      }
      event "X-Position", "Y-Position", "Z-Position": Value Change; "Move Stage": Mouse Up {
        n242 = event-data() -> ()  [unwired: 1 in, 3 out]
        n243 = local read "Workspace"() -> (w413:path)
        n244 = local read "Running"() -> (w415:bool)
        n245 = local read "PI SystemNumber"() -> (w408:i32)
        n246 = Not(x=w415) -> (.not. x?=w414:bool)
        n247 = Not Equal?(x=w413, y=path "") -> (x != y?=w411:bool)
        n248 = case shown="True" w411 {
          tunnel: w414 -> [_ w423]
          tunnel: w410 -> [_ w422]
          tunnel: [_ w421] -> w409
          tunnel: w408 -> [_ w420]
          tunnel: [_ w419] -> w405
          tunnel: [_ w418] -> w406
          tunnel: [_ w417] -> w407
          frame False {
            # "No Workspace Open"
            n249 = One Button Dialog(message="No Workspace Opened") -> ()  [unwired: 1 in, 1 out]
          }
          frame True {
            # "Move Stage if not Running"
            n250 = case shown="True" w423 {
              tunnel: w422 -> [_ w447]
              tunnel: [_ w437] -> w421
              tunnel: w420 -> [_ w445]
              tunnel: [_ w424] -> w419
              tunnel: [_ w425] -> w418
              tunnel: [_ w426] -> w417
              frame False {
              }
              frame True {
                w429 = 200
                n251 = local read "X-Position"() -> (w432:dbl)
                n252 = local read "Y-Position"() -> (w431:dbl)
                n253 = local read "Z-Position"() -> (w436:dbl)
                n254 = Subtract(x=w429, y=w432) -> (x-y=w433:dbl)
                n255 = Subtract(x=w429, y=w431) -> (x-y=w434:dbl)
                n256 = Subtract(x=w429, y=w436) -> (x-y=w435:dbl)
                n257 = Build Array(w433, w434, w435) -> (w446:dbl[])
                n258 = global read "GlobalConAxisPI.vi" "Conn. Axes"() -> (w444:string[])
                n259 = call "MOV.vi"("System no."=w445, "Axes to move"=w444, "Position values"=w446, "error in"=w447) -> ("error out"=w442:errorcluster)  [unwired: 15 in]
                n260 = call "POS?.vi"("System no."=w445, "Axes to query"=w444, "All axes?"=TRUE, "error in"=w442) -> ("Position"=w441:dbl[], "error out"=w437:errorcluster)  [unwired: 14 in]
                n261 = Index Array(array=w441, index #1=0 ("index"), index #2=1 ("index"), index #3=2 ("index")) -> (element #1=w430:dbl, element #2=w427:dbl, element #3=w428:dbl)
                n262 = Subtract(x=w429, y=w430) -> (x-y=w426:dbl)
                n263 = Subtract(x=w429, y=w427) -> (x-y=w425:dbl)
                n264 = Subtract(x=w429, y=w428) -> (x-y=w424:dbl)
              }
            }
          }
        }
        n265 = property on="y-position" class="DigNum (strict)"("Value"=w406) -> ()  [unwired: 2 in, 2 out]
        n266 = property on="z-position" class="DigNum (strict)"("Value"=w405) -> ()  [unwired: 2 in, 2 out]
        n267 = property on="x-position" class="DigNum (strict)"("Value"=w407) -> ()  [unwired: 2 in, 2 out]
      }
      event "Get Position": Value Change {
        w454 = 200
        n268 = event-data() -> ()  [unwired: 1 in, 5 out]
        n269 = local read "PI SystemNumber"() -> (w462:i32)
        n270 = global read "GlobalConAxisPI.vi" "Conn. Axes"() -> (w461:string[])
        n271 = call "POS?.vi"("System no."=w462, "Axes to query"=w461, "All axes?"=TRUE, "error in"=w463) -> ("Position"=w459:dbl[], "error out"=w455:errorcluster)  [unwired: 14 in]
        n272 = Index Array(array=w459, index #1=0 ("index"), index #2=1 ("index"), index #3=2 ("index")) -> (element #1=w451:dbl, element #2=w452:dbl, element #3=w453:dbl)
        n273 = Subtract(x=w454, y=w451) -> (x-y=w450:dbl)
        n274 = Subtract(x=w454, y=w452) -> (x-y=w449:dbl)
        n275 = Subtract(x=w454, y=w453) -> (x-y=w448:dbl)
        n276 = property on="y-position" class="DigNum (strict)"("Value"=w449) -> ()  [unwired: 2 in, 2 out]
        n277 = property on="x-position" class="DigNum (strict)"("Value"=w450) -> ()  [unwired: 2 in, 2 out]
        n278 = property on="z-position" class="DigNum (strict)"("Value"=w448) -> ()  [unwired: 2 in, 2 out]
      }
      event "New MSW": Mouse Up {
        # "Default Name"
        n279 = event-data() -> ()  [unwired: 1 in, 7 out]
        n280 = flat-sequence {
          tunnel: [w484] -> w467
          tunnel: w466 -> [w484]
          frame #0 {
            n281 = local write "Running"(TRUE ("MeasRunig")) -> ()
          }
        }
        n282 = Get Date/Time In Seconds() -> (seconds since 1Jan1904=w481:timestamp)
        n283 = Format Date/Time String(time format string (%c)="%Y-%m-%d", seconds (now)=w481) -> (date/time string=w479:string)  [unwired: 1 out]
        n284 = Concatenate Strings(w479, ".msw" ("string")) -> (w477:string)
        n285 = call "File Dialog"("start path"=path "D:/", "prompt"="Create New Workspace", "button label"="Create", "default name"=w477, "error in"=w467, "pattern (all files)"="*.msw", "pattern label"="MT Scan Workspace") -> ("selected path"=w471:path, "cancelled"=w472:bool, "error out"=w470:errorcluster)  [unwired: 5 in, 1 out]
        n286 = case shown="False" w472 {
          tunnel: w471 -> [w490 _]
          tunnel: w470 -> [w496 w498]
          tunnel: [w488 w497] -> w465
          tunnel: w468 -> [w486 _]
          frame False {
            # "Create Empty Workspace"
            n287 = local write "Workspace"(w490) -> ()
            n288 = call "MTS_CreateWriteMSW.vi"("Rewrite"=TRUE, "error in (no error)"=w496, "Workspace Path"=w490) -> ("error out"=w489:errorcluster, "Created"=w493:string, "Comment (dup)"=w492:string, "Files in Workspace (dup)"=w491:T21)  [unwired: 5 in]
            n289 = call "MTS_Workspace.vi"("Workspace"=w490, "Operation"=T20."Set Workspace", "Created in"=w493, "New Comment"=w492, "Files in Workspace in"=w491) -> ("Files in Workspace"=w487:T22)  [unwired: 3 in, 3 out]
            n290 = call "MTS_BuildWSTree.vi"("error in"=w489, "Files in Workspace"=w487, "Tree Refnum"=w486) -> ("error out"=w488:errorcluster)  [unwired: 6 in, 2 out]
          }
          frame True {
            n291 = call <vilib>:"Clear Errors.vi"("error in (no error)"=w498) -> ("error out"=w497:errorcluster)  [unwired: 6 in]
          }
        }
        n292 = flat-sequence {
          tunnel: w465 -> [w482]
          tunnel: [w482] -> w464
          frame #0 {
            n293 = local write "Running"(FALSE ("MeasRunig")) -> ()
          }
        }
      }
      event "Open MSW": Mouse Up {
        n294 = event-data() -> ()  [unwired: 1 in, 7 out]
        n295 = flat-sequence {
          tunnel: w502 -> [w514]
          tunnel: [w514] -> w501
          frame #0 {
            n296 = local write "Running"(TRUE ("MeasRunig")) -> ()
          }
        }
        n297 = call "File Dialog2"("start path"=path "D:/", "prompt"="Create New Workspace", "button label"="Open", "error in"=w501, "pattern (all files)"="*.msw", "pattern label"="MT Scan Workspace") -> ("selected path"=w506:path, "cancelled"=w507:bool, "error out"=w505:errorcluster)  [unwired: 6 in, 1 out]
        n298 = case shown="False" w507 {
          tunnel: w506 -> [w522 _]
          tunnel: w505 -> [w527 w529]
          tunnel: [w520 w528] -> w500
          tunnel: w503 -> [w519 _]
          frame False {
            # "Open Workspace"
            n299 = local write "Workspace"(w522) -> ()
            n300 = call "MTS_ReadMSW.vi"("error in (no error)"=w527, "Workspace Path"=w522) -> ("error out"=w521:errorcluster, "Created"=w525:string, "Comment"=w524:string, "Files in Workspace"=w523:T23)  [unwired: 6 in]
            n301 = call "MTS_Workspace.vi"("Workspace"=w522, "Operation"=T20."Set Workspace", "Created in"=w525, "New Comment"=w524, "Files in Workspace in"=w523) -> ("Files in Workspace"=w518:T22)  [unwired: 3 in, 3 out]
            n302 = Array To Cluster(array=w518) -> (cluster=w517:T24)
            n303 = Unbundle By Name(w517) -> ()  [unwired: 1 out]
            n304 = call "MTS_BuildWSTree.vi"("error in"=w521, "Files in Workspace"=w518, "Tree Refnum"=w519) -> ("error out"=w520:errorcluster, "numberOfFilesInWorkspace"=w516:i32)  [unwired: 6 in, 1 out]
            n305 = local write "Last Image File No"(w516) -> ()
          }
          frame True {
            n306 = call <vilib>:"Clear Errors.vi"("error in (no error)"=w529) -> ("error out"=w528:errorcluster)  [unwired: 6 in]
          }
        }
        n307 = flat-sequence {
          tunnel: w500 -> [w512]
          tunnel: [w512] -> w499
          frame #0 {
            n308 = local write "Running"(FALSE ("MeasRunig")) -> ()
          }
        }
      }
      event "Image": Mouse Up {
        w532 = 100.0 ("y")
        n309 = event-data() -> ("Coords"=w544:T25, "PlatMods"=w545:T26)  [unwired: 1 in, 5 out]
        n310 = invoke on="Image" class="IntGraph (strict)" method="Map Coords To XY"("Coords"=w544) -> ("Map Coords To XY"=w541:bool, "XY"=w539:cluster{"X":dbl, "Y":dbl})  [unwired: 6 in, 5 out]
        n311 = Unbundle By Name(w545) -> ("Ctrl"=w542:bool)
        n312 = And(x=w541, y=w542) -> (x .and. y?=w543:bool)
        n313 = Unbundle(w539) -> ("X"=w538:dbl, "Y"=w535:dbl)
        n314 = Multiply(x=w538, y=w532) -> (x*y=w537:dbl)
        n315 = Multiply(x=w535, y=w532) -> (x*y=w534:dbl)
        n316 = Round To Nearest(number=w537) -> (nearest integer value=w536:dbl)
        n317 = Round To Nearest(number=w534) -> (nearest integer value=w533:dbl)
        n318 = Divide(x=w536, y=w532) -> (x/y=w531:dbl)
        n319 = Divide(x=w533, y=w532) -> (x/y=w530:dbl)
        n320 = local read "Axis"() -> (w540:enum32{"x-y", "x-z", "y-x", "y-z", "z-x", "z-y"})
        n321 = case shown="True" w543 {
          tunnel: w540 -> [_ w548]
          tunnel: w531 -> [_ w547]
          tunnel: w530 -> [_ w546]
          frame False {
          }
          frame True {
            n322 = case shown="\"x-y\", Default" w548 {
              tunnel: w547 -> [w550 w552 w554]
              tunnel: w546 -> [w549 w551 w553]
              frame "x-y", Default {
                n323 = local write "X-Position"(w550) -> ()
                n324 = local write "Y-Position"(w549) -> ()
              }
              frame "x-z" {
                n325 = local write "X-Position"(w552) -> ()
                n326 = local write "Z-Position"(w551) -> ()
              }
              frame "y-z" {
                n327 = local write "Y-Position"(w554) -> ()
                n328 = local write "Z-Position"(w553) -> ()
              }
            }
          }
        }
      }
      event "WS File Tree": Value Change {
        n329 = event-data() -> ("NewVal"=w563:string)  [unwired: 1 in, 4 out]
        n330 = control-ref of="Workspace"() -> (w560:refnum<vi>)
        n331 = control-ref of="Histogram"() -> (w558:refnum<vi>)
        n332 = control-ref of="Trace"() -> (w557:refnum<vi>)
        n333 = control-ref of="Image"() -> (w556:refnum<vi>)
        n334 = control-ref of="Image"() -> (w555:refnum<vi>)
        n335 = control-ref of="Active pt3"() -> (w559:refnum<vi>)
        n336 = call "CreateNewWSfile.vi"("reference 5"=w555, "NewVal"=w563, "Image"=w556, "reference in"=w559, "error in (no error)"=w562, "reference 4"=w557, "reference 3"=w558, "Path in"=w560) -> ("error out"=w561:errorcluster)  [unwired: 3 in]
      }
      event "Resolution", "Picture size", "Pixel time", "Picture size 2", "Axis", "Laser  Profile": Value Change {
        n337 = event-data() -> ()  [unwired: 1 in, 5 out]
        n338 = local read "Axis"() -> (w584:enum32{"x-y", "x-z", "y-x", "y-z", "z-x", "z-y"})
        n339 = local read "Picture size"() -> (w586:dbl)
        n340 = local read "Resolution"() -> (w578:dbl)
        n341 = local read "X-Position"() -> (w581:dbl)
        n342 = local read "Y-Position"() -> (w580:dbl)
        n343 = local read "Z-Position"() -> (w579:dbl)
        n344 = local read "Pixel time"() -> (w587:dbl)
        n345 = local write "Axis"(w584) -> ()
        n346 = local read "Laser  Profile"() -> (w568:string)
        n347 = local read "Picture size 2"() -> (w585:dbl)
        n348 = local write "Pixel time"(w587) -> ()
        n349 = call "PI_CheckScan.vi"("Picture size"=w586, "Picture size 2"=w585, "Axis"=w584, "x-Position"=w581, "y-Position"=w580, "z-Position"=w579) -> ("Picture size out"=w582:dbl, "Picture size out 2"=w583:dbl)  [unwired: 8 in, 4 out]
        n350 = String To Byte Array(string=w568) -> (unsigned byte array=w566:u8[])
        n351 = local write "Picture size"(w582) -> ()
        n352 = local write "Picture size 2"(w583) -> ()
        n353 = Divide(x=w582, y=w578) -> (x/y=w590:dbl)
        n354 = Divide(x=w583, y=w578) -> (x/y=w591:dbl)
        n355 = Array Size(array=w566) -> (size(s)=w565:i32)
        n356 = Subtract(x=w566, y=48) -> (x-y=w572:i32[])
        n357 = Round Toward +Infinity(x=w590) -> (ceil(x): smallest int >= x=→"x":dbl)
        n358 = Round Toward +Infinity(x=w591) -> (ceil(x): smallest int >= x=→"y":dbl)
        n359 = Initialize Array(4, w565) -> (w576:i32[])
        n360 = Initialize Array(1, w565) -> (w574:i32[])
        n361 = In Range and Coerce(upper limit=w576, x=w572, lower limit=w574) -> (coerced(x)=w569:i32[])  [unwired: 1 out]
        n362 = Add(x=w569, y=48) -> (x+y=w571:i32[])
        n363 = Byte Array To String(unsigned byte array=w571) -> (string=w567:string)
        n364 = while {
          shift-right: [w596] -> w564
          shift-left: w567 -> [w600]
          i -> [w592]
          stop <- w595 stop-if-true
          n365 = Increment(x=w592) -> (x+1=w593:i32)
          n366 = String Subset(string=w600, offset (0)=w592, length (rest)=1) -> (substring=w598:string)
          n367 = Search and Replace String(replace all?=TRUE, input string=w600, search string=w598, offset=w593) -> (result string=w596:string)  [unwired: 4 in, 3 out]
          n368 = String Length(string=w596) -> (length=w594:i32)
          n369 = Less?(x=w594, y=w592) -> (x < y?=w595:bool)
        }
        n370 = local write "Laser  Profile"(w564) -> ()
      }
      event "SCANNER EMERGENCY": Value Change {
        n371 = event-data() -> ()  [unwired: 1 in, 5 out]
        n372 = local read "PI SystemNumber"() -> (w603:i32)
        n373 = call "PI Send String.vi"("System no."=w603, "String to send"="0RT", "error in"=w602) -> ("error out"=w605:errorcluster)  [unwired: 16 in]
        n374 = flat-sequence {
          tunnel: [w606] -> w601
          tunnel: w605 -> [w606]
          frame #0 {
            n375 = One Button Dialog(message="Emergency scanner stop appeared!!!\nCheck scanner settings before continue!!!") -> ()  [unwired: 2 out]
          }
        }
      }
      event "SET CCD": Value Change {
        n376 = event-data() -> ()  [unwired: 1 in, 6 out]
        n377 = call "Camera CCD Chip settings"("error in (no error)"=w609) -> ("Horizontal Binning"=w610:dbl, "Vertical Binning"=w615:dbl, "CCD Chip Horizontal Start"=w614:dbl, "CCD Chip Horizontal End"=w612:dbl, "CCD Chip Vertical Start"=w613:dbl, "CCD Chip Vertical End"=w611:dbl, "OK"=w616:bool, "error out"=w608:errorcluster)  [unwired: 11 in]
        n378 = case shown="True" w616 {
          tunnel: w615 -> [_ w624]
          tunnel: w614 -> [_ w623]
          tunnel: w613 -> [_ w622]
          tunnel: w612 -> [_ w621]
          tunnel: w611 -> [_ w620]
          tunnel: w610 -> [_ w619]
          tunnel: [_ w618] -> _
          tunnel: w608 -> [_ w617]
          frame False {
          }
          frame True {
            n379 = flat-sequence {
              tunnel: w624 -> [w631]
              tunnel: w623 -> [w625]
              tunnel: w622 -> [w630]
              tunnel: w621 -> [w629]
              tunnel: w620 -> [w628]
              tunnel: w619 -> [w627]
              tunnel: [w626] -> w618
              tunnel: w617 -> [w626]
              frame #0 {
                n380 = global write "GlobalSetGetConfigureCamera.vi" "Vbin"(w631) -> ()
                n381 = global write "GlobalSetGetConfigureCamera.vi" "Hbin"(w627) -> ()
                n382 = global write "ccdChipPixels.vi" "CCD Chip Vertical Start"(w630) -> ()
                n383 = Subtract(x=w629, y=w625) -> (x-y=w633:dbl)
                n384 = Subtract(x=w628, y=w630) -> (x-y=w632:dbl)
                n385 = global write "ccdChipPixels.vi" "CCD Chip horizontal start"(w625) -> ()
                n386 = global write "ccdChipPixels.vi" "CCD Chip Vertical end"(w628) -> ()
                n387 = global write "ccdChipPixels.vi" "CCD Chip horizontal end"(w629) -> ()
                n388 = Increment(x=w633) -> (x+1=w635:dbl)
                n389 = Increment(x=w632) -> (x+1=w634:dbl)
                n390 = Multiply(x=w635, y=w634) -> (x*y=w636:dbl)
                n391 = global write "ccdChipPixels.vi" "CCD Chip Size"(w636) -> ()
              }
            }
          }
        }
      }
      event "Set Temperature": Value Change {
        n392 = event-data() -> ()  [unwired: 1 in, 6 out]
        n393 = call "camera cooling"("error in (no error)"=w638) -> ("Temperature"=w639:dbl, "OK"=w640:bool, "error out"=w637:errorcluster)  [unwired: 16 in]
        n394 = case shown="True" w640 {
          tunnel: w639 -> [_ w644]
          tunnel: w637 -> [w641 w643]
          tunnel: [w641 w642] -> _
          frame False {
          }
          frame True {
            n395 = call "CheckTemperature.vi"("error in (no error)"=w643, "temperature in"=w644) -> ("error out"=w642:errorcluster)  [unwired: 9 in]
          }
        }
      }
      event "Cam (Defocused)": Value Change {
        n396 = event-data() -> ()  [unwired: 1 in, 6 out]
        n397 = global write "CamDef.vi" "CamDef"(w645) -> ()
      }
      event "OPEN SHUTER": Value Change {
        n398 = event-data() -> ()  [unwired: 1 in, 6 out]
        n399 = case shown="False" w647 {
          tunnel: [Shutter_mode_typedef."Close" ("mode") Shutter_mode_typedef."Open" ("mode")] -> w651
          tunnel: w648 -> [w653 w654]
          tunnel: [w653 w654] -> w650
          frame False {
          }
          frame True {
          }
        }
        n400 = call "SetShutter.vi"("type"=Shutter_type_typedef."TTL Low", "mode"=w651, "error in (no error)"=w650) -> ("error out"=w646:errorcluster)  [unwired: 11 in, 1 out]
      }
      event "Close": Value Change {
        n401 = event-data() -> ()  [unwired: 1 in, 6 out]
        n402 = case shown="True" w656 {
          tunnel: [Shutter_mode_typedef."Open" ("mode") Shutter_mode_typedef."Open" ("mode")] -> w660
          tunnel: w657 -> [w662 w663]
          tunnel: [w662 w663] -> w659
          frame False {
          }
          frame True {
          }
        }
        n403 = call "SetShutter.vi"("type"=Shutter_type_typedef."TTL Low", "mode"=w660, "error in (no error)"=w659) -> ()  [unwired: 11 in, 2 out]
      }
      event "Exposure": Value Change {
        n404 = event-data() -> ()  [unwired: 1 in, 6 out]
        n405 = call "Camera kinetic settings"("error in (no error)"=w668) -> ("Exposure time"=w665:dbl, "OK"=w666:bool, "error out"=w667:errorcluster)  [unwired: 16 in]
        n406 = case shown="True" w666 {
          tunnel: w665 -> [_ w669]
          frame False {
          }
          frame True {
            n407 = global write "GlobalSetGetConfigureCamera.vi" "Exposure"(w669) -> ()
          }
        }
      }
      event "Gain": Value Change {
        n408 = event-data() -> ()  [unwired: 1 in, 6 out]
        n409 = call "set gain"("error in (no error)"=w670) -> ("gain"=w672:dbl, "OK"=w671:bool)  [unwired: 16 in, 1 out]
        n410 = case shown="True" w671 {
          tunnel: w672 -> [_ w673]
          frame False {
          }
          frame True {
            n411 = global write "GlobalSetGetConfigureCamera.vi" "gain"(w673) -> ()
          }
        }
      }
      event "Start": Value Change {
        n412 = event-data() -> ()  [unwired: 1 in, 6 out]
        n413 = global write "GetPicture.vi" "GetPicture"(TRUE ("GetPicture")) -> ()
      }
      event "Measurement Time": Value Change {
        n414 = event-data() -> ()  [unwired: 1 in, 6 out]
        n415 = global write "GlobalSetGetConfigureCamera.vi" "Exposure"(w675) -> ()
      }
      event "Stop": Value Change {
        n416 = event-data() -> ()  [unwired: 1 in, 6 out]
        n417 = global write "StopGetPic.vi" "Stop"(TRUE ("Stop")) -> ()
      }
      event "Stop Program": Value Change {
        n418 = event-data() -> ()  [unwired: 1 in, 6 out]
        n419 = flat-sequence {
          tunnel: w677 -> [w681]
          tunnel: [w681] -> w680
          frame #0 {
            n420 = local write "Global Stop"(TRUE ("Global Stop")) -> ()
          }
        }
        n421 = local read "PI SystemNumber"() -> (w679:i32)
        n422 = call "Close connection if open.vi"("System no."=w679, "error in"=w680) -> ("error out"=w678:errorcluster)  [unwired: 16 in, 1 out]
      }
    }
    "z-position" <- w234
    "y-position" <- w218
    "x-position" <- w233
  }
  n423 = case shown="True" FALSE {
    tunnel: w7 -> [_ w683]
    frame False {
    }
    frame True {
      n424 = while {
        shift-right: [w687] -> _
        shift-left: w683 -> [w688]
        stop <- w685 stop-if-true
        n425 = Wait (ms)(milliseconds to wait=u32 100) -> ()  [unwired: 1 out]
        n426 = local read "Global Stop"() -> (w685:bool)
        n427 = control-ref of="CCD"() -> (w684:refnum<vi>)
        n428 = call "RunCameraPreview.vi"("error in (no error)"=w688, "CCD 3"=w684) -> ("error out"=w687:errorcluster)  [unwired: 9 in]
      }
    }
  }
  n429 = case shown="True" FALSE {
    tunnel: w7 -> [_ w689]
    frame False {
    }
    frame True {
      n430 = while {
        tunnel: w689 -> [w706]
        stop <- w692 stop-if-true
        n431 = local read "Global Stop"() -> (w707:bool)
        n432 = local read "Global Stop"() -> (w692:bool)
        n433 = call "Vision Acquisition"("Auto Exposure::Mode"="Auto Exposure::Mode", "Auto Exposure::Value"="Auto Exposure::Value", "Brightness::Mode"="Brightness::Mode", "Brightness::Value"="Brightness::Value", "Gain::Mode"="Gain::Mode", "Stop (F)"=w707, "Gain::Value"="Gain::Value", "error in"=w706, "Gamma::Mode"="Gamma::Mode", "Shutter::Mode"="Shutter::Mode", "Shutter::Value"="Shutter::Value", "Trigger::Trigger Activation"="Trigger::Trigger Activation", "Trigger::Trigger Mode"="Trigger::Trigger Mode", "Trigger::Trigger Parameter"="Trigger::Trigger Parameter", "Trigger Delay::Mode"="Trigger Delay::Mode") -> ("Image Out"=→"Image Out":T5, "Image Number"=→"Image Number":u32, "Frame Rate"=→"acquired FPS":dbl)  [unwired: 8 in, 2 out]
      }
    }
  }
  n434 = while {
    shift-right: [w715] -> w6
    shift-left: w7 -> [w712]
    shift-right: [w717] -> _
    shift-left: w7 -> [w722]
    tunnel: w15 -> [w716]
    tunnel: "Image Measurent Parameters" -> [w711]
    tunnel: [w710] -> _
    tunnel: "Sample description" -> [w709]
    stop <- w720 stop-if-true
    n435 = case shown="No Error" w712 {
      selector: w712 -> [w728 w1569]
      tunnel: w722 -> [w738 w1571]
      tunnel: [w737 TRUE ("Global Stop")] -> w719
      tunnel: [w733 w1571] -> w718
      tunnel: w716 -> [w732 _]
      tunnel: [w731 w1569] -> w715
      tunnel: [w729 T27."No Measurement" ("Do Measurement")] -> w713
      tunnel: w711 -> [w726 _]
      tunnel: [w725 w1569] -> w710
      tunnel: w709 -> [w723 _]
      frame No Error {
        n436 = while {
          shift-right: [w1567] -> w734
          shift-left: w738 -> [w1567]
          tunnel: [w1562] -> w736
          tunnel: [w1564] -> w735
          tunnel: [w1563] -> w730
          stop <- w1568 stop-if-true
          w1563 = FALSE ("FiFo Overrun")
          # "Wait for Start"
          n437 = local read "Task"() -> (w1562:T10)
          n438 = Wait (ms)(milliseconds to wait=u32 100) -> ()  [unwired: 1 out]
          n439 = local write "Stop Measurement"(w1563) -> ()
          n440 = local read "Global Stop"() -> (w1564:bool)
          n441 = Greater Than 0?(x=w1562) -> (x > 0?=w1566:bool)
          n442 = Or(x=w1566, y=w1564) -> (x .or. y?=w1568:bool)
        }
        n443 = control-ref of="WS File Tree"() -> (w727:refnum<vi>)
        n444 = case shown="\"Aquire Image\"" w736 {
          selector: w736 -> [_ _ w1097 _ _ _]
          tunnel: w728 -> [w739 w788 w1030 w1262 w1331 w1525]
          tunnel: [w739 w758 w1050 w1251 w1329 w1525] -> w731
          tunnel: [w740 FALSE ("Global Stop") FALSE ("Global Stop") FALSE ("Global Stop") FALSE ("Global Stop") FALSE ("Global Stop")] -> w737
          tunnel: w735 -> [w740 _ _ _ _ _]
          tunnel: w734 -> [w742 w772 w1115 w1261 w1330 w1526]
          tunnel: [w742 w772 w1120 w1261 w1330 w1524] -> w733
          tunnel: w732 -> [_ w838 w1052 _ _ _]
          tunnel: [T27."No Measurement" ("Do Measurement") T27."No Measurement" ("Do Measurement") w1096 T27."No Measurement" ("Do Measurement") T18."No Measurement" ("Do Measurement") w1523] -> w729
          tunnel: w727 -> [_ _ w1085 _ _ _]
          tunnel: w726 -> [_ w816 _ _ _ _]
          tunnel: [w739 w790 w1076 w1251 _ _] -> w725
          tunnel: "Laser pulse duration" -> [_ _ w1058 _ _ _]
          tunnel: w723 -> [_ _ w1049 _ _ _]
          frame "No Measurement", Default {
          }
          frame "Aquire Image" {
            w751 = 200
            w782 = T35."Image File" ("Measurement Type")
            w819 = 32768 ("dimension size")
            # "TODO:\n- FIFO Read Flag Buffer Half Full?\n- auto square pixels"
            # "Image Intensity Array"
            n445 = local read "PI SystemNumber"() -> (w760:i32)
            n446 = Index Array(array=w838) -> (element=w837:T36)  [unwired: 1 in]
            n447 = control-ref of="WS File Tree"() -> (w822:refnum<vi>)
            n448 = local read "Workspace"() -> (w827:path)
            n449 = local read "X-Position"() -> (w750:dbl)
            n450 = local read "Y-Position"() -> (w749:dbl)
            n451 = local read "Z-Position"() -> (w748:dbl)
            n452 = Unbundle By Name(w837) -> ("Dev"=w810:i32)
            n453 = Index Array(array=string[] ["yx", "yz", "xy", "xz", "zy", "zx"] ("Array"), index="Axis") -> (element=w765:string)
            n454 = Initialize Array(u32 0, w819) -> (w831:u32[])
            n455 = control-ref of="Image"() -> (w804:refnum<vi>)
            n456 = String To Byte Array(string="Laser  Profile") -> (unsigned byte array=w767:u8[])
            n457 = Subtract(x=w767, y=48) -> (x-y=w766:i32[])
            n458 = Initialize Array(0, 5, 2) -> (w764:i32[][])
            n459 = stacked-sequence {
              seq-local: [w857 _] -> [_ w884]
              seq-local: [w856 _] -> [_ w885]
              seq-local: [w855 _] -> [_ w880]
              seq-local: [w852 _] -> [_ w878]
              seq-local: [w851 _] -> [_ w877]
              seq-local: [w850 _] -> [_ w876]
              seq-local: [w849 _] -> [_ w872]
              tunnel: "Picture size" -> [w870 _]
              tunnel: "Picture size 2" -> [w869 _]
              tunnel: w816 -> [w868 _]
              tunnel: "X-Position" -> [w867 _]
              tunnel: "Y-Position" -> [w866 _]
              tunnel: "Z-Position" -> [w865 _]
              tunnel: "Axis" -> [w859 _]
              tunnel: "Resolution" -> [w855 _]
              tunnel: [w858 _] -> w744
              tunnel: [_ w886] -> w789
              tunnel: w788 -> [w853 _]
              tunnel: w765 -> [_ w883]
              tunnel: "Laser  Profile" -> [_ w882]
              tunnel: "Pixel time" -> [w854 w881]
              tunnel: w760 -> [_ w879]
              tunnel: [_ w871] -> w785
              tunnel: [_ w875] -> w784
              tunnel: [_ w874] -> w783
              tunnel: [_ w873] -> w775
              frame #0 {
                n460 = call "PI_CheckScan.vi"("Picture size"=w870, "Picture size 2"=w869, "Axis"=w859, "x-Position"=w867, "y-Position"=w866, "z-Position"=w865, "error in (no error)"=w853) -> ("error out"=w849:errorcluster, "Picture size out"=w856:dbl, "Picture size out 2"=w857:dbl, "a0"=w852:dbl, "b0"=w851:dbl, "c0"=w850:dbl)  [unwired: 7 in]
                n461 = Divide(x=w856, y=w855) -> (x/y=w862:dbl)
                n462 = Divide(x=w857, y=w855) -> (x/y=w863:dbl)
                n463 = local write "Picture size"(w856) -> ()
                n464 = local write "Picture size 2"(w857) -> ()
                n465 = Round Toward +Infinity(x=w862) -> (ceil(x): smallest int >= x=w861:dbl)
                n466 = Round Toward +Infinity(x=w863) -> (ceil(x): smallest int >= x=w860:dbl)
                n467 = Bundle("a0"=w852, "b0"=w851, "c0"=w850) -> (w864:cluster{"a0":dbl, "b0":dbl, "c0":dbl})  [unwired: 1 in]
                n468 = Bundle By Name(cluster=w868, "Position"=w864, "Axis 1 Pixels"=w861, "Axis 2 Pixels"=w860, "Axis"=w859, "Resolution"=w855, "PixelTime"=w854) -> (w858:T8)
              }
              frame #1 {
                n469 = call "PI_AreaScan_Prepare_1.vi"("System"=w879, "Laser"=w882, "Axis"=w883, "da"=w885, "db"=w884, "error in (no error)"=w872, "a0"=w878, "b0"=w877, "Resolution"=w880, "c0"=w876, "Pixel time"=w881) -> ("Tacq"=w871:dbl, "lp"=w874:i32, "ap"=w875:i32, "Trigger"=w873:dbl[], "error out"=w886:errorcluster)  [unwired: 4 in]
                "Measure. time" <- w871
              }
            }
            n470 = Replace Array Subset(array=w764, new element=w766, index (col)=0) -> (w762:i32[][])  [unwired: 1 in]
            n471 = Unbundle By Name(w744) -> ("Axis 1 Pixels"=w797:dbl, "Axis 2 Pixels"=w798:dbl, "Resolution"=w795:dbl, "PixelTime"=w779:dbl)  [unwired: 2 out]
            n472 = Multiply(x=w785, y=1000) -> (x*y=w794:dbl)
            n473 = case shown="False" FALSE {
              tunnel: TRUE -> [_ w848]
              tunnel: [w842 w847] -> w790
              tunnel: w789 -> [w842 w846]
              tunnel: w784 -> [_ w845]
              tunnel: w783 -> [_ w844]
              tunnel: "Laser  Profile" -> [_ w843]
              frame False {
              }
              frame True {
                n474 = call "AOTF-Trigger_1.vi"("Channel"=w843, "error in (no error)"=w846, "Triggered"=w848, "lp"=w844, "ap"=w845) -> ("error out"=w847:errorcluster)  [unwired: 2 in]
              }
            }
            n475 = Divide(x=w779, y=1000) -> (x/y=w777:dbl)
            n476 = Divide(x=w797, y=w795) -> (x/y=w806:dbl)
            n477 = Divide(x=w798, y=w795) -> (x/y=w808:dbl)
            n478 = call "HH_Set.vi"("Device List"=w838, "CFD Settings"="CFD Settings", "error in (no error)"=w789, "SyncDiv"=8) -> ("ht3 header out"=w802:T37, "Sync Rate"=w800:i32, "error out"=w774:errorcluster)  [unwired: 7 in, 2 out]
            n479 = Round Toward +Infinity(x=w794) -> (ceil(x): smallest int >= x=w792:dbl)
            n480 = Round Toward +Infinity(x=w806) -> (ceil(x): smallest int >= x=w805:dbl)
            n481 = Round Toward +Infinity(x=w808) -> (ceil(x): smallest int >= x=w807:dbl)
            n482 = call "MTS_PreapareImage.vi"("WS File Tree"=w822, "Workspace"=w827, "Measurement Type"=w782, "Image Measurent Parameters"=w744, "error in"=w774, "Trigger"=w775) -> ("File Name (dup)"=w812:path, "File No"=→"Last Image File No":i32, "Image Header"=w814:T38, "Comment"=w815:string, "error out"=w773:errorcluster)  [unwired: 5 in]
            n483 = Divide(x=1024, y=w800) -> (x/y=w781:dbl)
            n484 = local write "Active pt3"(w812) -> ()
            n485 = call "Scan_SetGraphScales.vi"("error in (no error)"=w773, "Image Measurent Parameters"=w744, "Image"=w804) -> ("error out"=w803:errorcluster)  [unwired: 8 in]
            n486 = Initialize Array(0 ("element"), w805, w807) -> (w778:i32[][])
            n487 = call "HT3_Create.vi"("Laser"=w762, "Image Header in"=w814, "Save pt3"="Save Files", "Measurement Type"=w782, "error in"=w803, "Comment"=w815, "ht3 Header in"=w802, "File Path"=w812) -> ("error out"=w828:errorcluster, "FileHeaderPos"=w818:T39, "refnum out"=w826:refnum<file>)  [unwired: 1 in]
            n488 = call "HH_Start.vi"("Device Index"=w810, "Acq. Time"=w792, "error in (no error)"=w828) -> ("error out"=w835:errorcluster)  [unwired: 11 in, 1 out]
            n489 = Unbundle By Name(w835) -> ("status"=w836:bool)
            n490 = Not(x=w836) -> (.not. x?=w834:bool)
            n491 = case shown="True" w834 {
              tunnel: [w934 w965] -> w833
              tunnel: w760 -> [_ w960]
              tunnel: w835 -> [w935 w961]
              tunnel: w810 -> [w933 w952]
              tunnel: w778 -> [_ w937]
              tunnel: w831 -> [_ w959]
              tunnel: w819 -> [_ w958]
              tunnel: [w932 w957] -> w830
              tunnel: [w932 w956] -> w829
              tunnel: w826 -> [w931 w955]
              tunnel: [w931 w954] -> w825
              tunnel: [0 ("Num Records Total") w953] -> w824
              tunnel: [0.0 w946] -> w823
              tunnel: w765 -> [_ w949]
              tunnel: [dbl[] [] w943] -> w780
              tunnel: w777 -> [_ w939]
              tunnel: w775 -> [_ w938]
              frame False {
                (unwired) i32[][] [] ("Image Array Out")
                (unwired) u64[] [] ("Histograms")
                w932 = FALSE ("Stop Measurement")
                n492 = call "HH_Stop.vi"("Device Index"=w933, "error in (no error)"=w935) -> ("error out"=w934:errorcluster)  [unwired: 12 in, 1 out]
              }
              frame True {
                # "Overflow Interv. Time (s)"
                # "No Error"
                n493 = call "PI Start WG.vi"("System no."=w960, "axis"=w949, "Generator"=T28."both axis", "Init DDL"=T29."none", "increment"=T29."slow axis", "error in"=w961, "saved data"=T30."actual position") -> ("error out"=w962:errorcluster)  [unwired: 12 in]
                n494 = Initialize Array(0, 5) -> (w940:i32[])
                n495 = while {
                  tunnel: w952 -> [w985]
                  tunnel: w959 -> [w1001]
                  tunnel: w958 -> [w1000]
                  shift-right: [w986] -> w964
                  shift-left: w962 -> [w1002]
                  shift-right: [FALSE ("Reset")] -> _
                  shift-left: TRUE ("Reset") -> [w973]
                  tunnel: [w994] -> w957
                  tunnel: [w990] -> w956
                  tunnel: w955 -> [w992]
                  tunnel: [w991] -> w954
                  tunnel: [w969] -> w953
                  tunnel: [w968] -> w946
                  shift-right: [w982] -> w945
                  shift-left: w940 -> [w980]
                  tunnel: [w979] -> w944
                  tunnel: w939 -> [w976]
                  tunnel: w938 -> [_]
                  shift-right: [w967] -> w936
                  shift-left: w937 -> [w975]
                  i -> [w978]
                  stop <- w999 stop-if-true
                  n496 = call "HH_FIFORead.vi"("Device Index"=w985, "Buffer In"=w1001, "Count"=w1000, "error in (no error)"=w1002) -> ("OK"=w995:bool, "Buffer Out"=w972:u32[], "Data Count"=w971:i32, "FiFo Overrun"=w994:bool, "error out"=w993:errorcluster)  [unwired: 7 in]
                  n497 = local read "Global Stop"() -> (w988:bool)
                  n498 = local read "Stop Measurement"() -> (w989:bool)
                  n499 = local write "Buffer Overrun"(w994) -> ()
                  n500 = Unbundle(w993) -> ("status"=w998:bool)  [unwired: 2 out]
                  n501 = call "HT3_Write.vi"("error in"=w993, "Data Count"=w971, "Data in"=w972, "refnum in"=w992) -> ("error out"=w987:errorcluster, "refnum out"=w991:refnum<file>)  [unwired: 6 in]
                  n502 = call "GetCountRates.vi"("error in (no error)"=w987, "DeviceIndex"=w985) -> ("error out"=w986:errorcluster, "CntRates"=w984:dbl[], "SyncRate"=w977:i32)  [unwired: 1 in]
                  n503 = Or(x=w989, y=w988) -> (x .or. y?=w990:bool)
                  n504 = Multiply(x=w976, y=w977) -> (x*y=w966:dbl)
                  n505 = Compound Arithmetic op=OR(invert w995, w998, w988, w989) -> (w999:bool)
                  n506 = Insert Into Array(array=w984, index=0, new element=w977) -> (w981:dbl[])
                  n507 = call "HH_ToImage.vi"("Data In"=w972, "Reset"=w973, "Image Array In"=w975, "Data Count"=w971, "Pixel Time (Laser Pulses)"=w966) -> ("Image Array Out"=w967:i32[][], "Histograms"=→"Histogram":i32[][], "Total Oveflow Count"=w968:u64, "Num Records Total"=w969:i64, "Traces"=→"Trace":i32[][])  [unwired: 4 in, 2 out]
                  n508 = Add(x=w980, y=w981) -> (x+y=w982:dbl[])
                  n509 = Wait (ms)(milliseconds to wait=u32 2) -> ()  [unwired: 1 out]
                  n510 = Increment(x=w978) -> (x+1=w979:i32)
                }
                "Image" <- w936
                n511 = call "HH_Stop.vi"("Device Index"=w952, "error in (no error)"=w964) -> ("error out"=w965:errorcluster)  [unwired: 12 in, 1 out]
                n512 = Divide(x=w945, y=w944) -> (x/y=w943:dbl[])
              }
            }
            n513 = flat-sequence {
              tunnel: w833 -> [w905]
              tunnel: [w894] -> w759
              tunnel: w830 -> [w907]
              tunnel: w829 -> [w896]
              tunnel: w760 -> [w904]
              tunnel: [w903] -> w757
              tunnel: w825 -> [w901]
              tunnel: w824 -> [w900]
              tunnel: w823 -> [w890]
              tunnel: w818 -> [w895]
              tunnel: w781 -> [w891]
              tunnel: w780 -> [w887]
              frame #0 {
                # "Count Rate (per s)"
                # "Finish after Aquire Image"
                n514 = Or(x=w896, y=w907) -> (x .or. y?=w906:bool)
                n515 = Multiply(x=w891, y=w890) -> (x*y=w889:dbl)
                n516 = case shown="False" w906 {
                  tunnel: w905 -> [w912 w923]
                  tunnel: w904 -> [w910 w921]
                  tunnel: [w909 w921] -> w903
                  tunnel: [w911 w920] -> w902
                  tunnel: [enum16{"timeover", "manual", "overflow"}."timeover" ("Stop Reason") w926] -> w897
                  tunnel: w896 -> [w908 w924]
                  frame False {
                    # "Stop WaveGen\nif Aborted"
                    n517 = case shown="False" w908 {
                      tunnel: w912 -> [w914 w919]
                      tunnel: [w914 w916] -> w911
                      tunnel: w910 -> [w915 w917]
                      tunnel: [w915 w917] -> w909
                      frame False {
                      }
                      frame True {
                        n518 = call "PI Send String.vi"("System no."=w917, "String to send"="0RT", "error in"=w919) -> ("error out"=w916:errorcluster)  [unwired: 16 in]
                      }
                    }
                  }
                  frame True {
                    n519 = call "PI Send String.vi"("System no."=w921, "String to send"="0RT", "error in"=w923) -> ("error out"=w920:errorcluster)  [unwired: 16 in]
                    n520 = Select(t=enum16{"timeover", "manual", "overflow"}."manual" ("Stop Reason"), s=w924, f=enum16{"timeover", "manual", "overflow"}."overflow" ("Stop Reason")) -> (s? t:f=w926:enum16{"timeover", "manual", "overflow"})
                  }
                }
                n521 = Multiply(x=w889, y=1000.0) -> (x*y=w899:dbl)
                n522 = property on="Aquire Image" class="Bool"("BoolText.Text"="Aquire Image" ("Caption.Text"), "BoolText.TextColor"=u32 0 ("Boolean Text.Colors:FG Color")) -> ()  [unwired: 2 in, 2 out]
                n523 = To Long Integer(number=w899) -> (32bit integer=w898:i32)
                n524 = call "HT3_Finish.vi"("FileHeaderPos"=w895, "Rates"=w887, "Stop Reason"=w897, "error in"=w902, "Num Records"=w900, "Stop After (ms)"=w898, "refnum in"=w901) -> ("error out"=w894:errorcluster)  [unwired: 4 in]
              }
            }
            n525 = global read "GlobalConAxisPI.vi" "Conn. Axes"() -> (w756:string[])
            n526 = Subtract(x=w751, y=w750) -> (x-y=w747:dbl)
            n527 = Subtract(x=w751, y=w749) -> (x-y=w746:dbl)
            n528 = Subtract(x=w751, y=w748) -> (x-y=w745:dbl)
            n529 = Build Array(w747, w746, w745) -> (w755:dbl[])
            n530 = call "MOV.vi"("System no."=w757, "Axes to move"=w756, "Position values"=w755, "error in"=w759) -> ("error out"=w758:errorcluster)  [unwired: 15 in]
          }
          frame "Point Measurement", "Auto Point" {
            w1012 = 200
            w1019 = 200
            w1053 = 0
            w1083 = 32768 ("dimension size")
            n531 = local read "PI SystemNumber"() -> (w1027:i32)
            n532 = Index Array(array=w1052) -> (element=w1125:T36)  [unwired: 1 in]
            n533 = local read "Workspace"() -> (w1113:path)
            n534 = local read "X-Position"() -> (w1103:dbl)
            n535 = local read "Y-Position"() -> (w1102:dbl)
            n536 = local read "Z-Position"() -> (w1031:dbl)
            n537 = Unbundle By Name(w1125) -> ("Dev"=w1038:i32)
            n538 = Initialize Array(u32 0, w1083) -> (w1118:u32[])
            n539 = local read "concatenated string"() -> (w1045:string)
            n540 = local read "Last Image File No"() -> (w1089:i32)
            n541 = local read "CFD Settings"() -> (w1078:T7)
            n542 = local read "Laser  Profile"() -> (w1067:string)
            n543 = Not(x="Adjustment") -> (.not. x?=w1047:bool)
            n544 = Equal?(x=w1097, y=T10."Auto Point" ("Task")) -> (x = y?=w1032:bool)
            n545 = And(x=w1032, y="Autopoint-Autofocus Z") -> (x .and. y?=w1084:bool)
            n546 = String Length(string=w1067) -> (length=w1057:i32)
            n547 = String To Byte Array(string=w1067) -> (unsigned byte array=w1065:u8[])
            n548 = Select(t="AutoPoint" ("Measurement Type"), s=w1032, f="Point" ("Measurement Type")) -> (s? t:f=w1044:string)
            n549 = Select(t=w1089, s=w1032, f=-1) -> (s? t:f=w1087:i32)
            n550 = case shown="False" FALSE {
              tunnel: [w1127 w1133] -> w1076
              tunnel: FALSE -> [_ w1132]
              tunnel: 5 -> [_ w1131]
              tunnel: w1067 -> [_ w1130]
              tunnel: w1058 -> [_ w1129]
              tunnel: w1030 -> [w1127 w1128]
              frame False {
              }
              frame True {
                n551 = call "AOTF-Trigger_1.vi"("Channel"=w1130, "Pulse length"=w1129, "Sync trigger ratio"=w1131, "error in (no error)"=w1128, "Triggered"=w1132) -> ("error out"=w1133:errorcluster)  [unwired: 2 in]
              }
            }
            n552 = Select(t="Auto Measurement Time (ms)", s=w1032, f="Measurement Time") -> (s? t:f=w1081:i32)
            n553 = Select(t=T31."Auto Point" ("Measurement Type"), s=w1032, f=T31."Point Measurement" ("Measurement Type")) -> (s? t:f=w1091:T31)
            n554 = Array Subset(array=w1058, index=w1053, length=w1057) -> (w1056:i32[])
            n555 = Subtract(x=w1065, y=48) -> (x-y=w1060:i32[])
            n556 = Select(t=T10."Auto Measurement Control" ("Task"), s=w1032, f=T27."No Measurement" ("Do Measurement")) -> (s? t:f=w1096:T10)
            n557 = Concatenate Strings(w1045, w1044) -> (w1043:string)
            n558 = Initialize Array(0, 5, 2) -> (w1061:i32[][])
            n559 = Multiply(x=w1081, y=1000) -> (x*y=w1080:i32)
            n560 = Replace Array Subset(array=w1061, new element=w1060, index (col)=w1053) -> (w1059:i32[][])  [unwired: 1 in]
            n561 = local read "Pattern"() -> (w1040:dbl[][])
            n562 = local read "NxtAutMesPoint"() -> (w1039:i32)
            n563 = Bundle("X-Position"=w1103, "Y-Position"=w1102, "Z-Position"=w1031) -> (w1086:T16)  [unwired: 1 in]
            n564 = Replace Array Subset(array=w1059, new element=w1056, index (col)=1) -> (w1055:i32[][])  [unwired: 1 in]
            n565 = call "MTS_AutoPointCords.vi"("Is Auto Point"=w1032, "Cords In"=w1086, "Next Auto Measure Point"=w1039, "Pattern"=w1040) -> ("Cords"=w1071:T16)  [unwired: 7 in]
            n566 = global read "GlobalConAxisPI.vi" "Conn. Axes"() -> (w1021:string[])
            n567 = Unbundle By Name(w1071) -> ("X-Position"=w1018:dbl, "Y-Position"=w1016:dbl, "Z-Position"=w1013:dbl)
            n568 = call "MTS_GenFileComment.vi"("Measurement Type"=w1091, "Parent File No"=w1087, "Info"=w1049, "Upper Left"=w1071, "error in"=w1115) -> ("Comment"=w1114:string, "error out"=w1112:errorcluster)  [unwired: 7 in, 2 out]
            n569 = Subtract(x=w1019, y=w1013) -> (x-y=w1014:dbl)
            n570 = Subtract(x=w1019, y=w1016) -> (x-y=w1015:dbl)
            n571 = Subtract(x=w1019, y=w1018) -> (x-y=w1017:dbl)
            n572 = Build Array(w1017, w1015, w1014) -> (w1020:dbl[])
            n573 = call "MOV.vi"("System no."=w1027, "Axes to move"=w1021, "Position values"=w1020, "error in"=w1030) -> ("error out"=w1029:errorcluster)  [unwired: 15 in]
            n574 = call "POS?.vi"("System no."=w1027, "Axes to query"=w1021, "All axes?"=TRUE, "error in"=w1029) -> ("Position"=w1025:dbl[], "error out"=w1028:errorcluster)  [unwired: 14 in]
            n575 = Index Array(array=w1025, index #1=0 ("index"), index #2=1 ("index"), index #3=2 ("index")) -> (element #1=w1011:dbl, element #2=w1010:dbl, element #3=w1009:dbl)
            n576 = call "MTS_GetNextFileName.vi"("error in (no error)"=w1112, "File Type"="ht3", "Measurement Type"=w1043, "Workspace"=w1113) -> ("error out"=w1107:errorcluster, "Next File Name"=w1106:path)  [unwired: 6 in]
            n577 = case shown="True" w1047 {
              tunnel: w1107 -> [w1141 w1149]
              tunnel: w1106 -> [_ w1148]
              tunnel: [w1141 w1147] -> w1105
              tunnel: [path "D:/tmp.ht3" w1142] -> w1104
              tunnel: w1091 -> [_ w1144]
              tunnel: w1087 -> [_ w1146]
              tunnel: w1085 -> [_ w1143]
              frame False {
              }
              frame True {
                n578 = call "MTS_AddFileToWorkspace.vi"("File Name"=w1148, "File Type"=T32."pt3 File", "Measurement Type"=w1144, "error in (no error)"=w1149, "Parent"=w1146, "Tree Refnum"=w1143) -> ("File Name (dup)"=w1142:path, "error out"=w1147:errorcluster)  [unwired: 7 in, 1 out]
              }
            }
            n579 = Subtract(x=w1012, y=w1009) -> (x-y=w1006:dbl)
            n580 = Subtract(x=w1012, y=w1010) -> (x-y=w1007:dbl)
            n581 = Subtract(x=w1012, y=w1011) -> (x-y=w1008:dbl)
            n582 = call "HH_Set.vi"("Device List"=w1052, "CFD Settings"=w1078, "error in (no error)"=w1028) -> ("ht3 header out"=w1101:T37, "Sync Rate"=w1068:i32, "error out"=w1099:errorcluster)  [unwired: 8 in, 2 out]
            n583 = property on="x-position" class="DigNum (strict)"("Value"=w1008) -> ()  [unwired: 2 in, 2 out]
            n584 = property on="z-position" class="DigNum (strict)"("Value"=w1006) -> ()  [unwired: 2 in, 2 out]
            n585 = property on="y-position" class="DigNum (strict)"("Value"=w1007) -> ()  [unwired: 2 in, 2 out]
            n586 = Bundle By Name(cluster=w1101, "AcquisitionTime (ms)"=w1080) -> (w1100:T37)
            n587 = Divide(x=65536 ("n"), y=w1068) -> (x/y=w1069:dbl)
            n588 = case shown="True" w1084 {
              tunnel: w1099 -> [w1150 w1158]
              tunnel: [w1150 w1157] -> w1098
              tunnel: w1027 -> [_ w1152]
              tunnel: w1069 -> [_ w1156]
              tunnel: w1071 -> [_ w1155]
              tunnel: w1038 -> [_ w1151]
              frame False {
              }
              frame True {
                # "Auto Z"
                n589 = call "MTS_AutoZPos.vi"("PH Dev"=w1151, "OFlow Interv [s]"=w1156, "PI System no."=w1152, "error in"=w1158, "Start Point"=w1155) -> ("New Z"=w1154:dbl, "Counts"=→"Counts":u32[], "error out"=w1157:errorcluster)  [unwired: 7 in, 1 out]
                n590 = local write "Z-Position"(w1154) -> ()
              }
            }
            n591 = call "HT3_Create.vi"("Laser"=w1055, "Save pt3"=w1047, "error in"=w1098, "Comment"=w1114, "ht3 Header in"=w1100, "File Path"=w1104) -> ("error out"=w1036:errorcluster, "FileHeaderPos"=w1082:T39, "refnum out"=w1110:refnum<file>)  [unwired: 3 in]
            n592 = case shown="False" w1032 {
              tunnel: [w1135 w1139] -> w1035
              tunnel: w1036 -> [w1136 w1137]
              tunnel: "Auto Defocussed Cam" -> [_ w1138]
              tunnel: "Point Defocussed Cam" -> [w1134 _]
              frame False {
                n593 = property on="3dAbelFcs" class="Bool (strict)"(error in=w1136, "Value"=w1134) -> (error out=w1135:errorcluster)  [unwired: 1 in, 1 out]
              }
              frame True {
                n594 = property on="3dAbelFcs" class="Bool (strict)"(error in=w1137, "Value"=w1138) -> (error out=w1139:errorcluster)  [unwired: 1 in, 1 out]
              }
            }
            n595 = call "HH_Start.vi"("Device Index"=w1038, "Acq. Time"=w1080, "error in (no error)"=w1036) -> ("error out"=w1034:errorcluster)  [unwired: 11 in, 1 out]
            n596 = Unbundle By Name(w1034) -> ("status"=w1124:bool)
            n597 = Merge Errors(w1034, w1035) -> (w1033:errorcluster)
            n598 = Not(x=w1124) -> (.not. x?=w1123:bool)
            n599 = case shown="True" w1123 {
              tunnel: [w1193 w1216] -> w1121
              tunnel: w1033 -> [w1194 w1204]
              tunnel: w1105 -> [w1195 w1215]
              tunnel: [w1195 w1214] -> w1122
              tunnel: w1038 -> [w1188 w1203]
              tunnel: w1118 -> [_ w1211]
              tunnel: w1083 -> [_ w1210]
              tunnel: [w1192 w1209] -> w1117
              tunnel: [w1192 w1208] -> w1116
              tunnel: w1110 -> [w1191 w1207]
              tunnel: [w1191 w1206] -> w1109
              tunnel: [i64 0 ("Num Records Total") w1205] -> w1108
              tunnel: [dbl[] [] w1200] -> w1073
              tunnel: [0 w1199] -> w1072
              frame False {
                w1192 = FALSE ("Stop Measurement")
                n600 = call "HH_Stop.vi"("Device Index"=w1188, "error in (no error)"=w1194) -> ("error out"=w1193:errorcluster)  [unwired: 12 in, 1 out]
              }
              frame True {
                # "Overflow Interv. Time (s)"
                # "No Error"
                n601 = Initialize Array(0, 5) -> (w1198:i32[])
                n602 = while {
                  tunnel: w1203 -> [w1225]
                  tunnel: w1211 -> [w1249]
                  tunnel: w1210 -> [w1248]
                  shift-right: [w1226] -> w1213
                  shift-left: w1204 -> [w1250]
                  shift-right: [w1247] -> w1214
                  shift-left: w1215 -> [w1247]
                  shift-right: [FALSE ("Reset")] -> _
                  shift-left: TRUE ("Reset") -> [w1243]
                  tunnel: [w1240] -> w1209
                  tunnel: [w1232] -> w1208
                  tunnel: w1207 -> [w1236]
                  tunnel: [w1235] -> w1206
                  tunnel: [w1234] -> w1205
                  tunnel: [w1233] -> w1199
                  shift-right: [w1220] -> w1201
                  shift-left: w1198 -> [w1219]
                  tunnel: [w1217] -> w1202
                  i -> [w1218]
                  stop <- w1246 stop-if-true
                  n603 = call "HH_FIFORead.vi"("Device Index"=w1225, "Buffer In"=w1249, "Count"=w1248, "error in (no error)"=w1250) -> ("OK"=w1241:bool, "Buffer Out"=w1237:u32[], "Data Count"=w1238:i32, "FiFo Overrun"=w1240:bool, "error out"=w1239:errorcluster)  [unwired: 7 in]
                  n604 = Wait (ms)(milliseconds to wait=u32 10) -> ()  [unwired: 1 out]
                  n605 = local read "Global Stop"() -> (w1230:bool)
                  n606 = local write "Buffer Overrun"(w1240) -> ()
                  n607 = Unbundle(w1239) -> ("status"=w1245:bool)  [unwired: 2 out]
                  n608 = call "HT3_Write.vi"("error in"=w1239, "Data Count"=w1238, "Data in"=w1237, "refnum in"=w1236) -> ("error out"=w1227:errorcluster, "refnum out"=w1235:refnum<file>)  [unwired: 6 in]
                  n609 = local read "Stop Measurement"() -> (w1231:bool)
                  n610 = call "HH_TraceAndHisto.vi"("Data In"=w1237, "Reset"=w1243, "Data Count"=w1238) -> ("Histograms"=w1229:i32[][], "Total Oveflow Count"=w1233:u64, "Num Records Total"=w1234:i64, "Traces"=w1228:i32[][])  [unwired: 8 in, 1 out]
                  n611 = local write "Trace"(w1228) -> ()
                  n612 = call "GetCountRates.vi"("error in (no error)"=w1227, "DeviceIndex"=w1225) -> ("error out"=w1226:errorcluster, "CntRates"=w1221:dbl[], "SyncRate"=w1222:i32)  [unwired: 1 in]
                  n613 = Or(x=w1231, y=w1230) -> (x .or. y?=w1232:bool)
                  n614 = Compound Arithmetic op=OR(invert w1241, w1245, w1230, w1231) -> (w1246:bool)
                  n615 = local write "Histogram"(w1229) -> ()
                  n616 = Insert Into Array(array=w1221, index=0, new element=w1222) -> (w1223:dbl[])
                  n617 = Add(x=w1219, y=w1223) -> (x+y=w1220:dbl[])
                  n618 = Increment(x=w1218) -> (x+1=w1217:i32)
                }
                n619 = Divide(x=w1201, y=w1202) -> (x/y=w1200:dbl[])
                n620 = call "HH_Stop.vi"("Device Index"=w1203, "error in (no error)"=w1213) -> ("error out"=w1216:errorcluster)  [unwired: 12 in, 1 out]
              }
            }
            n621 = flat-sequence {
              tunnel: w1122 -> [w1179]
              tunnel: w1121 -> [w1175]
              tunnel: [w1179] -> w1120
              tunnel: [w1172] -> w1051
              tunnel: w1117 -> [w1177]
              tunnel: w1116 -> [w1168]
              tunnel: w1109 -> [w1171]
              tunnel: w1108 -> [w1170]
              tunnel: w1082 -> [w1167]
              tunnel: w1073 -> [w1164]
              tunnel: w1072 -> [w1163]
              frame #0 {
                # "Finish after Measurement"
                n622 = Or(x=w1168, y=w1177) -> (x .or. y?=w1176:bool)
                n623 = Index Array(array=w1164, index=0) -> (element=w1165:dbl)
                n624 = case shown="False" w1176 {
                  tunnel: w1175 -> [w1181 w1182]
                  tunnel: [w1181 w1182] -> w1173
                  tunnel: [enum16{"timeover", "manual", "overflow"}."timeover" ("Stop Reason") w1185] -> w1169
                  tunnel: w1168 -> [_ w1183]
                  frame False {
                  }
                  frame True {
                    n625 = Select(t=enum16{"timeover", "manual", "overflow"}."manual" ("Stop Reason"), s=w1183, f=enum16{"timeover", "manual", "overflow"}."overflow" ("Stop Reason")) -> (s? t:f=w1185:enum16{"timeover", "manual", "overflow"})
                  }
                }
                n626 = Divide(x=w1163, y=w1165) -> (x/y=w1162:dbl)
                n627 = Multiply(x=1024000, y=w1162) -> (x*y=w1160:dbl)
                n628 = To Long Integer(number=w1160) -> (32bit integer=w1159:i32)
                n629 = property on="Point Measurement" class="Bool"("BoolText.Text"="Point Measurement" ("Caption.Text"), "BoolText.TextColor"=u32 0 ("Boolean Text.Colors:FG Color")) -> ()  [unwired: 2 in, 2 out]
                n630 = call "HT3_Finish.vi"("FileHeaderPos"=w1167, "Rates"=w1164, "Stop Reason"=w1169, "error in"=w1173, "Num Records"=w1170, "Stop After (ms)"=w1159, "refnum in"=w1171) -> ("error out"=w1172:errorcluster)  [unwired: 4 in]
              }
            }
            n631 = call "MOV.vi"("System no."=w1027, "Axes to move"=w1021, "Position values"=w1020, "error in"=w1051) -> ("error out"=w1050:errorcluster)  [unwired: 15 in]
          }
          frame "Save Color Image" {
            n632 = control-ref of="WS File Tree"() -> (w1259:refnum<vi>)
            n633 = local read "Active pt3"() -> (w1258:path)
            n634 = call "MTS_GetFileFromWS.vi"(".pt3 File Name"=w1258) -> ("File Header"=w1257:T40)  [unwired: 9 in, 1 out]
            n635 = Unbundle By Name(w1257) -> ("Measurement Type"=w1256:T41, "Pixels"=w1253:i32[])
            n636 = Equal?(x=T31."Image File" ("Measurement Type"), y=w1256) -> (x = y?=w1254:bool)
            n637 = case shown="True" w1254 {
              tunnel: w1262 -> [w1263 w1286]
              tunnel: w1258 -> [_ w1285]
              tunnel: w1258 -> [_ _]
              tunnel: [w1263 w1265] -> w1251
              tunnel: w1259 -> [_ _]
              tunnel: w1253 -> [_ w1270]
              frame False {
              }
              frame True {
                # "Image Intensity Array"
                # "Image Intensity Array"
                n638 = call "HT3_Open.vi"("error in"=w1286, "File Path"=w1285) -> ("error out"=w1278:errorcluster, "Header"=w1282:T42, "refnum out"=w1284:refnum<file>)  [unwired: 3 in, 4 out]
                n639 = Index Array(array=w1270, index #2=1 ("index")) -> (element #1=w1267:i32, element #2=w1268:i32)  [unwired: 1 in]
                n640 = Unbundle By Name(w1282) -> ()  [unwired: 15 out]
                n641 = Initialize Array(0 ("element"), w1267, w1268) -> (w1280:i32[][])
                n642 = Initialize Array(0 ("element"), 4 ("dimension size"), w1267, w1268) -> (w1273:i32[][][])
                n643 = while {
                  tunnel: w1284 -> [w1311]
                  shift-right: [FALSE ("Start From Top")] -> _
                  shift-left: TRUE ("Start From Top") -> [w1305]
                  shift-right: [w1304] -> w1277
                  shift-left: w1278 -> [w1302]
                  tunnel: [w1303] -> w1276
                  tunnel: w1280 -> [w1301]
                  tunnel: [w1300] -> w1279
                  tunnel: [w1301] -> _
                  stop <- w1308 stop-if-true
                  n644 = call "HT3_Read.vi"("Start From Top"=w1305, "error in"=w1302, "Data count"=10000, "refnum in"=w1311) -> ("error out"=w1304:errorcluster, "Data out"=w1307:u32[], "refnum out"=w1303:refnum<file>, "EOF?"=w1308:bool)  [unwired: 4 in]
                  n645 = Array Size(array=w1307) -> (size(s)=w1306:i32)
                  n646 = call "HH_FileToImage_1.vi"("Data In"=w1307, "Reset"=w1305, "Data Count"=w1306) -> ("Histograms"=w1300:i32[][])  [unwired: 7 in, 5 out]
                }
                n647 = call "MTS_SelectTCSPCBinning.vi"("Histograms in"=w1279) -> ("TCSPC Binning"=w1272:i32[][])  [unwired: 1 in, 9 out]
                n648 = while {
                  tunnel: w1276 -> [w1299]
                  shift-right: [FALSE ("Start From Top")] -> _
                  shift-left: TRUE ("Start From Top") -> [w1293]
                  shift-right: [w1292] -> w1264
                  shift-left: w1277 -> [w1288]
                  tunnel: [w1291] -> w1266
                  tunnel: w1273 -> [w1290]
                  tunnel: [w1289] -> _
                  tunnel: w1272 -> [w1287]
                  stop <- w1296 stop-if-true
                  n649 = call "HT3_Read.vi"("Start From Top"=w1293, "error in"=w1288, "Data count"=10000, "refnum in"=w1299) -> ("error out"=w1292:errorcluster, "Data out"=w1295:u32[], "refnum out"=w1291:refnum<file>, "EOF?"=w1296:bool)  [unwired: 4 out]
                  n650 = Array Size(array=w1295) -> (size(s)=w1294:i32)
                  n651 = call "HH_ToColorImage.vi"("Data In"=w1295, "Reset"=w1293, "Image Array In"=w1290, "Data Count"=w1294, "TCSPC Binning"=w1287) -> ("Image Array Out"=w1289:i32[][][])  [unwired: 2 in, 8 out]
                }
                n652 = Close File(refnum=w1266, error in=w1264) -> (error out=w1265:errorcluster)  [unwired: 1 out]
              }
            }
          }
          frame "Find Single Mol." {
            # "dirty trick"
            n653 = local read "Active pt3"() -> (w1338:path)
            n654 = local read "Picture size"() -> (w1322:dbl)
            n655 = local read "Picture size 2"() -> (w1319:dbl)
            n656 = local read "Y-Position"() -> (w1312:dbl)
            n657 = local read "X-Position"() -> (w1313:dbl)
            n658 = local read "Resolution"() -> (w1320:dbl)
            n659 = Divide(x=w1322, y=w1320) -> (x/y=w1321:dbl)
            n660 = Divide(x=w1319, y=w1320) -> (x/y=w1318:dbl)
            n661 = call "MTS_GetFileFromWS.vi"(".pt3 File Name"=w1338) -> ("File Header"=w1337:T40)  [unwired: 9 in, 1 out]
            n662 = Unbundle By Name(w1337) -> ("Measurement Type"=w1336:T41, "Pixels"=w1324:i32[], "Upper Left"=w1333:T43, "Scan Axis"=w1332:enum32{"x-y", "x-z", "y-z"})
            n663 = Build Array(w1322, w1319) -> (w1328:dbl[])
            n664 = Equal?(x=T31."Image File" ("Measurement Type"), y=w1336) -> (x = y?=w1334:bool)
            n665 = call "MTS_ScannerXYZToImageXY.vi"("Axis"=w1332, "Scanner XYZ"=w1333) -> ("Image Y"=w1315:dbl, "Image X"=w1317:dbl)
            n666 = case shown="True" TRUE {
              tunnel: [w1341 w1344] -> w1323
              tunnel: w1324 -> [w1341 _]
              tunnel: w1321 -> [_ w1348]
              tunnel: w1318 -> [_ w1347]
              tunnel: [w1340 w1343] -> w1316
              tunnel: w1317 -> [w1340 _]
              tunnel: [w1339 w1342] -> w1314
              tunnel: w1315 -> [w1339 _]
              tunnel: w1313 -> [_ w1343]
              tunnel: w1312 -> [_ w1342]
              frame False {
              }
              frame True {
                n667 = To Long Integer(number=w1348) -> (32bit integer=w1346:i32)
                n668 = To Long Integer(number=w1347) -> (32bit integer=w1345:i32)
                n669 = Build Array(w1346, w1345) -> (w1344:i32[])
              }
            }
            n670 = case shown="True" w1334 {
              tunnel: w1331 -> [w1349 w1416]
              tunnel: w1338 -> [_ _]
              tunnel: w1338 -> [_ _]
              tunnel: [w1349 w1421] -> w1329
              tunnel: w1323 -> [_ w1439]
              tunnel: w1328 -> [_ w1420]
              tunnel: w1316 -> [_ w1431]
              tunnel: w1314 -> [_ w1432]
              frame False {
              }
              frame True {
                w1385 = T11 1 items=["Center of Mass X", "Center of Mass Y", "First Pixel X", "First Pixel Y", "Bounding Rect Left", "Bounding Rect Top", "Bounding Rect Right", "Bounding Rect Bottom", "Max Feret Diameter Start X", "Max Feret Diameter Start Y", "Max Feret Diameter End X", "Max Feret Diameter End Y", "Max Horiz. Segment Length Left", "Max Horiz. Segment Length Right", "Max Horiz. Segment Length Row", "-", "Bounding Rect Width", "Bounding Rect Height", "Bounding Rect Diagonal", "Perimeter", "Convex Hull Perimeter", "Holes' Perimeter", "Max Feret Diameter", "Equivalent Ellipse Major Axis", "Equivalent Ellipse Minor Axis", "Equivalent Ellipse Minor Axis (Feret)", "Equivalent Rect Long Side", "Equivalent Rect Short Side", "Equivalent Rect Diagonal", "Equivalent Rect Short Side (Feret)", "Average Horiz. Segment Length", "Average Vert. Segment Length", "Hydraulic Radius", "Waddel Disk Diameter", "-", "Area", "Holes' Area", "Particle & Holes' Area", "Convex Hull Area", "Image Area", "-", "Number of Holes", "Number of Horiz. Segments", "Number of Vert. Segments", "-", "Orientation", "Max Feret Diameter Orientation", "-", "% Area/Image Area", "% Area/(Particle & Holes' Area)", "Ratio of Equivalent Ellipse Axes", "Ratio of Equivalent Rect Sides", "-", "Elongation Factor", "Compactness Factor", "Heywood Circularity Factor", "Type Factor", "-", "Sum X", "Sum Y", "Sum XX", "Sum XY", "Sum YY", "Sum XXX", "Sum XXY", "Sum XYY", "Sum YYY", "-", "Moment of Inertia XX", "Moment of Inertia XY", "Moment of Inertia YY", "Moment of Inertia XXX", "Moment of Inertia XXY", "Moment of Inertia XYY", "Moment of Inertia YYY", "Norm. Moment of Inertia XX", "Norm. Moment of Inertia XY", "Norm. Moment of Inertia YY", "Norm. Moment of Inertia XXX", "Norm. Moment of Inertia XXY", "Norm. Moment of Inertia XYY", "Norm. Moment of Inertia YYY", "Hu Moment 1", "Hu Moment 2", "Hu Moment 3", "Hu Moment 4", "Hu Moment 5", "Hu Moment 6", "Hu Moment 7"] ("Measurement Parameter")
                w1366 = TRUE ("Measurement Type")
                w1390 = T11 0 items=["Center of Mass X", "Center of Mass Y", "First Pixel X", "First Pixel Y", "Bounding Rect Left", "Bounding Rect Top", "Bounding Rect Right", "Bounding Rect Bottom", "Max Feret Diameter Start X", "Max Feret Diameter Start Y", "Max Feret Diameter End X", "Max Feret Diameter End Y", "Max Horiz. Segment Length Left", "Max Horiz. Segment Length Right", "Max Horiz. Segment Length Row", "-", "Bounding Rect Width", "Bounding Rect Height", "Bounding Rect Diagonal", "Perimeter", "Convex Hull Perimeter", "Holes' Perimeter", "Max Feret Diameter", "Equivalent Ellipse Major Axis", "Equivalent Ellipse Minor Axis", "Equivalent Ellipse Minor Axis (Feret)", "Equivalent Rect Long Side", "Equivalent Rect Short Side", "Equivalent Rect Diagonal", "Equivalent Rect Short Side (Feret)", "Average Horiz. Segment Length", "Average Vert. Segment Length", "Hydraulic Radius", "Waddel Disk Diameter", "-", "Area", "Holes' Area", "Particle & Holes' Area", "Convex Hull Area", "Image Area", "-", "Number of Holes", "Number of Horiz. Segments", "Number of Vert. Segments", "-", "Orientation", "Max Feret Diameter Orientation", "-", "% Area/Image Area", "% Area/(Particle & Holes' Area)", "Ratio of Equivalent Ellipse Axes", "Ratio of Equivalent Rect Sides", "-", "Elongation Factor", "Compactness Factor", "Heywood Circularity Factor", "Type Factor", "-", "Sum X", "Sum Y", "Sum XX", "Sum XY", "Sum YY", "Sum XXX", "Sum XXY", "Sum XYY", "Sum YYY", "-", "Moment of Inertia XX", "Moment of Inertia XY", "Moment of Inertia YY", "Moment of Inertia XXX", "Moment of Inertia XXY", "Moment of Inertia XYY", "Moment of Inertia YYY", "Norm. Moment of Inertia XX", "Norm. Moment of Inertia XY", "Norm. Moment of Inertia YY", "Norm. Moment of Inertia XXX", "Norm. Moment of Inertia XXY", "Norm. Moment of Inertia XYY", "Norm. Moment of Inertia YYY", "Hu Moment 1", "Hu Moment 2", "Hu Moment 3", "Hu Moment 4", "Hu Moment 5", "Hu Moment 6", "Hu Moment 7"] ("Measurement Parameter")
                w1410 = T44 4 items=["Grayscale (U8)", "Grayscale (I16)", "Grayscale (SGL)", "Complex (CSG)", "RGB (U32)", "HSL (U32)", "RGB (U64)", "Grayscale (U16)"] ("Image Type")
                w1418 = T44 4 items=["Grayscale (U8)", "Grayscale (I16)", "Grayscale (SGL)", "Complex (CSG)", "RGB (U32)", "HSL (U32)", "RGB (U64)", "Grayscale (U16)"] ("Image Type")
                w1438 = 1 ("index")
                # "Gauss Width"
                # "Pixel Size [um]"
                n671 = local read "Image"() -> (w1399:i32[][])
                n672 = Array To Cluster(array=T34 [] ("MesaurementSelection")) -> (cluster=w1393:T45)
                n673 = Unbundle By Name(w1393) -> ("MesaurementSelection[0]"=w1391:T46, "MesaurementSelection[1]"=w1386:T46, "MesaurementSelection[2]"=w1381:T46, "MesaurementSelection[3]"=w1372:T46)
                n674 = Random Number (0-1)() -> (number: 0 to 1=w1409:dbl)
                n675 = Random Number (0-1)() -> (number: 0 to 1=w1415:dbl)
                n676 = Number To Decimal String(number=w1409) -> (decimal integer string=w1408:string)  [unwired: 1 in]
                n677 = Number To Decimal String(number=w1415) -> (decimal integer string=w1414:string)  [unwired: 1 in]
                n678 = Concatenate Strings(w1414, "IMAQ CreatePatternimg" ("Image Name")) -> (w1412:string)
                n679 = Concatenate Strings(w1408, "IMAQ CreatePatternimg2" ("Image Name")) -> (w1406:string)
                n680 = call "IMAQ Create"("Image Name"=w1412, "Image Type"=w1418, "error in (no error)"=w1416) -> ("New Image"=w1417:T5, "error out"=w1401:errorcluster)  [unwired: 2 in]
                n681 = Bundle By Name(cluster=w1372, "Measurement Parameter"="Measurement Parameter 2", "Range Lower Value"="Range Lower Value Par 2", "Range Upper Value"="Range Upper Value Par 2", "Range"="Ex/In Par 2", "Measurement Type"=w1366) -> (w1371:T46)
                n682 = Bundle By Name(cluster=w1391, "Measurement Parameter"=w1390, "Range Lower Value"="X Start 2", "Range Upper Value"="X End 2", "Range"="Exclude / Include X", "Measurement Type"=w1366) -> (w1380:T46)
                n683 = Bundle By Name(cluster=w1386, "Measurement Parameter"=w1385, "Range Lower Value"="Y Start 2", "Range Upper Value"="Y End 2", "Range"="Exclude / Include Y", "Measurement Type"=w1366) -> (w1379:T46)
                n684 = Bundle By Name(cluster=w1381, "Measurement Parameter"="Measurement Parameter 1", "Range Lower Value"="Range Lower Value Par 1", "Range Upper Value"="Range Upper Value  Par 1", "Range"="Ex/In Par 1", "Measurement Type"=w1366) -> (w1378:T46)
                n685 = Build Array(w1380, w1379, w1378, w1371) -> (w1377:T34)
                n686 = call "MTS_IntensityArrayToImage.vi"(0:"Image"=w1417, 1:"Image"=w1399, "error in (no error)"=w1401, "Log Scale"=FALSE) -> ("Image Out"=w1365:T5, "error out"=w1357:errorcluster)  [unwired: 10 in]
                n687 = call "IMAQ Create"("Image Name"=w1406, "Image Type"=w1410, "error in (no error)"=w1357) -> ("New Image"=w1400:T5, "error out"=w1356:errorcluster)  [unwired: 2 in]
                n688 = call "MTS_IntensityArrayToImage.vi"(0:"Image"=w1400, 1:"Image"=w1399, "error in (no error)"=w1356, "Log Scale"=TRUE) -> ("Image Out"=w1350:T5, "error out"=w1355:errorcluster)  [unwired: 10 in]
                n689 = case shown="True" TRUE ("Forget all just match") {
                  tunnel: "Remove Outliers" -> [_ w1473]
                  tunnel: [w1444 w1463] -> w1411
                  tunnel: w1355 -> [w1449 w1472]
                  tunnel: [w1443 w1461] -> w1397
                  tunnel: "Filter" -> [_ w1471]
                  tunnel: w1377 -> [_ w1470]
                  tunnel: w1365 -> [w1450 w1465]
                  tunnel: path "C:/Users/Core-FCS/Desktop/Documents/AbelFCS/ParticleFinder/SingleMoleculePatternFinder/Patterns/azimutalGolden.png" ("Template File Path (GeometricMatching)") -> [w1448 _]
                  tunnel: "Settings (GeometricMatching)" -> [w1442 _]
                  tunnel: IMAQ_Rounding_Mode."Optimize" ("Rounding Mode Gaussian") -> [_ w1469]
                  tunnel: IMAQ_Rounding_Mode."Optimize" ("Rounding Mode Convolution") -> [_ w1468]
                  tunnel: "Square/Hexa" -> [_ w1467]
                  tunnel: "Connectivity 4/8" -> [_ w1466]
                  tunnel: w1350 -> [w1441 w1459]
                  tunnel: [w1441 w1456] -> w1354
                  tunnel: [w1440 w1457] -> w1352
                  frame False {
                    n690 = call "SingleMoleculePatternFinder.vi"("Image In"=w1450, "Settings (GeometricMatching)"=w1442, "error in"=w1449, "Template File Path (GeometricMatching)"=w1448) -> ("Matches (GeometricMatching)"=w1447:T47[], "Number of Matches (GeometricMatching)"=w1443:i32, "error out"=w1440:errorcluster)  [unwired: 21 in]
                    n691 = for {
                      N: w1443 -> [_]
                      tunnel: w1447 -> [w1455]
                      tunnel: [w1452] -> w1446 mode=indexing
                      tunnel: [w1451] -> w1445 mode=indexing
                      i -> [w1454]
                      n692 = Index Array(array=w1455, index=w1454) -> (element=w1453:T47)
                      n693 = Unbundle By Name(w1453) -> ("Position.x"=w1452:sgl, "Position.y"=w1451:sgl)
                    }
                    n694 = Build Array(w1446, w1445) -> (w1444:sgl[][])
                  }
                  frame True {
                    n695 = call "SingleMoleFinderEasy.vi"("Image Src"=w1465, "Number of Erosion"=w1473, "HolesBorder"=w1471, "Selection Values"=w1470, "Rounding Mode Gaussian"=w1469, "error in"=w1472, "Rounding Mode Convolution"=w1468, "Square/Hexa (Square)"=w1467, "Connectivity 4/8 (8)"=w1466) -> ("Number of Particles"=w1460:i32, "Particle Measurements (Pixels)"=w1462:dbl[][], "error out"=w1458:errorcluster)  [unwired: 15 in, 1 out]
                    n696 = case shown="True" "Manual" {
                      tunnel: w1458 -> [w1477 w1485]
                      tunnel: [w1477 w1484] -> w1457
                      tunnel: [w1474 w1483] -> w1456
                      tunnel: [w1475 w1482] -> w1463
                      tunnel: w1462 -> [w1475 w1479]
                      tunnel: [w1476 w1481] -> w1461
                      tunnel: w1460 -> [w1476 w1480]
                      tunnel: w1459 -> [w1474 w1478]
                      frame False {
                      }
                      frame True {
                        n697 = while {
                          tunnel: w1485 -> [w1500]
                          tunnel: [w1499] -> w1484
                          tunnel: w1478 -> [w1498]
                          tunnel: [w1497] -> w1483
                          shift-right: [w1490] -> w1482
                          shift-left: w1479 -> [w1489]
                          tunnel: [w1488] -> w1481
                          tunnel: w1480 -> [w1487]
                          i -> [w1494]
                          stop <- w1496 stop-if-true
                          n698 = call "IMAQ Select Point"("Window Number (0...15)"=1, "error in (no error)"=w1500, "Image In"=w1498) -> ("error out"=w1499:errorcluster, "Cancelled"=w1496:bool, "Point"=w1495:T48, "Image Out (duplicate)"=w1497:T5)  [unwired: 5 in]
                          n699 = Unbundle(w1495) -> ("X"=w1493:sgl, "Y"=w1492:sgl)
                          n700 = Build Array(w1493, w1492) -> (w1491:sgl[])
                          n701 = Add(x=w1487, y=w1494) -> (x+y=w1488:i32)
                          n702 = Insert Into Array(array=w1489, index (row)=w1488, new element=w1491) -> (w1490:dbl[][])  [unwired: 1 in]
                        }
                      }
                    }
                  }
                }
                "Number of Particles" <- w1397
                n703 = Index Array(array=w1439, index #2=w1438) -> (element #1=w1436:i32, element #2=w1435:i32)  [unwired: 1 in]
                n704 = Index Array(array=w1420, index #2=w1438) -> (element #1=w1437:dbl, element #2=w1434:dbl)  [unwired: 1 in]
                n705 = Divide(x=w1437, y=w1436) -> (x/y=w1428:dbl)
                n706 = Divide(x=w1434, y=w1435) -> (x/y=w1433:dbl)
                n707 = Index Array(array=w1411, index (col) #1=0 ("index (row)"), index (col) #2=1 ("index (col)")) -> (element #1=w1403:dbl[], element #2=w1405:dbl[])  [unwired: 2 in]
                n708 = To Word Integer(number=w1403) -> (16bit integer=w1402:i16[])
                n709 = To Word Integer(number=w1405) -> (16bit integer=w1404:i16[])
                n710 = Multiply(x=w1428, y=w1402) -> (x*y=w1430:dbl[])
                n711 = Multiply(x=w1404, y=w1433) -> (x*y=w1429:dbl[])
                n712 = Add(x=w1431, y=w1430) -> (x+y=w1424:dbl[])
                n713 = Add(x=w1429, y=w1432) -> (x+y=w1423:dbl[])
                n714 = Build Array(w1424, w1423, w1402, w1404) -> (→"Pattern":dbl[][])
                n715 = for {
                  N: w1397 -> [_]
                  shift-right: [w1507] -> w1353
                  shift-left: w1354 -> [w1508]
                  tunnel: w1402 -> [w1506] mode=indexing
                  tunnel: w1404 -> [w1505] mode=indexing
                  shift-right: [w1509] -> w1351
                  shift-left: w1352 -> [w1510]
                  tunnel: u32 16738560 -> [w1504]
                  tunnel: 3.0 ("x") -> [w1503]
                  n716 = call "MTS_DrawCrossIMAQIamge.vi"("Image"=w1508, "Size"=w1503, "Color"=w1504, "X"=w1506, "Y"=w1505, "error in (no error)"=w1510) -> ("Image Out"=w1507:T5, "error out"=w1509:errorcluster)  [unwired: 8 in]
                }
                "AM image" <- w1353
                n717 = global write "patternImg.vi" "New Image"(w1353) -> ()
                n718 = flat-sequence {
                  tunnel: w1351 -> [w1502]
                  tunnel: [w1502] -> w1421
                  frame #0 {
                    n719 = local write "Tab Control"(T4."AutoMesaurement" ("Tab Control")) -> ()
                  }
                }
              }
            }
          }
          frame "Auto Measurement Control" {
            # "Init"
            n720 = local read "Pattern"() -> (w1521:dbl[][])
            n721 = Index Array(array=w1521, index (row) #1=2 ("index (row)"), index (row) #2=3 ("index (col)")) -> (element #1=w1518:dbl[], element #2=→"subarray":dbl[])  [unwired: 2 in]
            n722 = local read "NxtAutMesPoint"() -> (w1529:i32)
            n723 = Less Than 0?(x=w1529) -> (x < 0?=w1532:bool)
            n724 = Increment(x=w1529) -> (x+1=w1512:i32)
            "NxtAutMesPoint" <- w1512
            n725 = Array Size(array=w1518) -> (size(s)=w1517:i32)
            n726 = case shown="True" w1532 {
              tunnel: w1526 -> [w1553 w1557]
              tunnel: [w1553 w1556] -> w1530
              tunnel: [w1552 w1554] -> w1528
              tunnel: w1517 -> [_ w1554]
              frame False {
                n727 = local read "Auto Measure Points"() -> (w1552:i32)
              }
              frame True {
                n728 = Number To Decimal String(number=w1554) -> (decimal integer string=w1559:string)  [unwired: 1 in]
                n729 = Concatenate Strings("Point 1 / " ("Caption.Text"), w1559) -> (w1558:string)
                n730 = property on="Auto Meas Progress" class="Slide (strict)"(error in=w1557, "Scale.Minimum"=0.0 ("Scale.Range:Minimum"), "Scale.Maximum"=w1554, "Value"=1 ("Auto Meas Progress"), "Caption.Text"=w1558) -> (error out=w1556:errorcluster)  [unwired: 1 in, 1 out]
                "Auto Measure Points" <- w1554
              }
            }
            n731 = Increment(x=w1512) -> (x+1=w1527:i32)
            n732 = Index Array(array=w1521, index (row) #1=2 ("index (row)"), index (col) #1=w1512, index (row) #2=3 ("index (col)"), index (col) #2=w1512) -> (element #1=w1520:dbl, element #2=w1519:dbl)
            n733 = Greater Or Equal?(x=w1512, y=w1528) -> (x >= y?=w1531:bool)
            n734 = case shown="False" w1531 {
              tunnel: w1530 -> [w1543 w1551]
              tunnel: [w1549 w1551] -> w1524
              tunnel: [T18."Auto Point" ("Do Measurement") T18."No Measurement" ("Do Measurement")] -> w1523
              tunnel: w1527 -> [w1544 _]
              tunnel: w1520 -> [w1541 _]
              tunnel: w1519 -> [w1540 _]
              tunnel: w1528 -> [w1537 _]
              frame False {
                # "Prpare For Next Point"
                # "1 loc max  2 undef 0 saddle -1 local min"
                n735 = Number To Decimal String(number=w1544) -> (decimal integer string=w1546:string)  [unwired: 1 in]
                n736 = Number To Decimal String(number=w1537) -> (decimal integer string=w1538:string)  [unwired: 1 in]
                n737 = Concatenate Strings("Point " ("Caption.Text"), w1546, " / " ("Caption.Text"), w1538) -> (w1545:string)
                n738 = global read "patternImg.vi" "New Image"() -> (w1533:T5)
                n739 = call "MTS_DrawCrossIMAQIamge.vi"("Image"=w1533, "Size"=3.0 ("x"), "Color"=u32 6618880, "X"=w1541, "Y"=w1540, "error in (no error)"=w1543) -> ("Image Out"=w1534:T5, "error out"=w1542:errorcluster)  [unwired: 8 in]
                n740 = property on="Auto Meas Progress" class="Slide (strict)"(error in=w1542, "Value"=w1544, "Caption.Text"=w1545) -> (error out=w1549:errorcluster)  [unwired: 1 in, 1 out]
                n741 = local write "AM image"(w1534) -> ()
              }
              frame True {
                # "No More Points"
              }
            }
          }
        }
        n742 = local write "Buffer Overrun"(w730) -> ()
      }
      frame Error {
      }
    }
    n743 = local read "Global Stop"() -> (w721:bool)
    n744 = flat-sequence {
      tunnel: w718 -> [w1577]
      tunnel: [w1577] -> w717
      tunnel: w713 -> [w1574]
      frame #0 {
        n745 = local write "Task"(w1574) -> ()
        n746 = Equal?(x=w1574, y=T27."No Measurement" ("Do Measurement")) -> (x = y?=w1575:bool)
        n747 = Not(x=w1575) -> (.not. x?=w1576:bool)
        n748 = local write "Running"(w1576) -> ()
      }
    }
    n749 = Unbundle(w715) -> ("status"=w714:bool)  [unwired: 2 out]
    n750 = Compound Arithmetic op=OR(w714, w719, w721) -> (w720:bool)
  }
  n751 = global read "patternImg.vi" "New Image"() -> (w4:T5)
  n752 = call "IMAQ Dispose"("Image"=w4, "error in (no error)"=w6) -> ()  [unwired: 4 in, 1 out]
